vi "Entrenamiento Fuerza 5.vi"(8 "error in (no error)":errorcluster) -> (0 "error out":errorcluster)   [LabVIEW 2014]
panel:
  out "Label":string
  out "Master":bool
  out "element":T1
  in  "Master":bool
  out "OK":bool
  out "error out 2":errorcluster
  in  "Puerto Serial":refnum<visa-resource-name>="COM25"
  in  "index":i32
  out "size(s)":i32
  out "Decorations[]":refnum<vi>[](array[refnum])
  out "Boolean":bool
  out "Impulso":string
  out "Tiempo Restante":string
  out "Tiempo Transcurrido":string
  in  "Start":bool
  in  "Impulso":bool
  in  "Reset":bool
  in  "Back":bool
  in  "Help":bool
  in  "Slider":i32(slide) scale=0.0..100.0
  out "Horizontal Graduated Bar":i16(slide) scale=0.0..100.0
  in  "Remove Button":bool
  in  "Add Button":bool
  out "Opcional %":string="0%"
  in  "Opcional Bool":bool
  out "Biceps %":string="0%"
  in  "Biceps Bool":bool
  out "Pectorales %":string="0%"
  in  "Pectorales Bool":bool
  out "Trapecio %":string="0%"
  in  "Trapecio Bool":bool
  out "Dorsales %":string="0%"
  in  "Dorsales Bool":bool
  out "Lumbares %":string="0%"
  in  "Lumbares Bool":bool
  out "Abdomen %":string="0%"
  in  "Abdomen Bool":bool
  out "Gluteos %":string="0%"
  in  "Gluteos Bool":bool
  out "Isquiotibiales %":string="0%"
  in  "Isquiotibiales Bool":bool
  in  "Stop":bool
  out "Cuadríceps %":string="0%"
  in  "Cuadriceps Bool":bool
  out "date/time string":string="22/08/2015 01:25:29 a. m."
  # "Entrenamiento de Fuerza"
  # "Presentación"
  # "Seg"
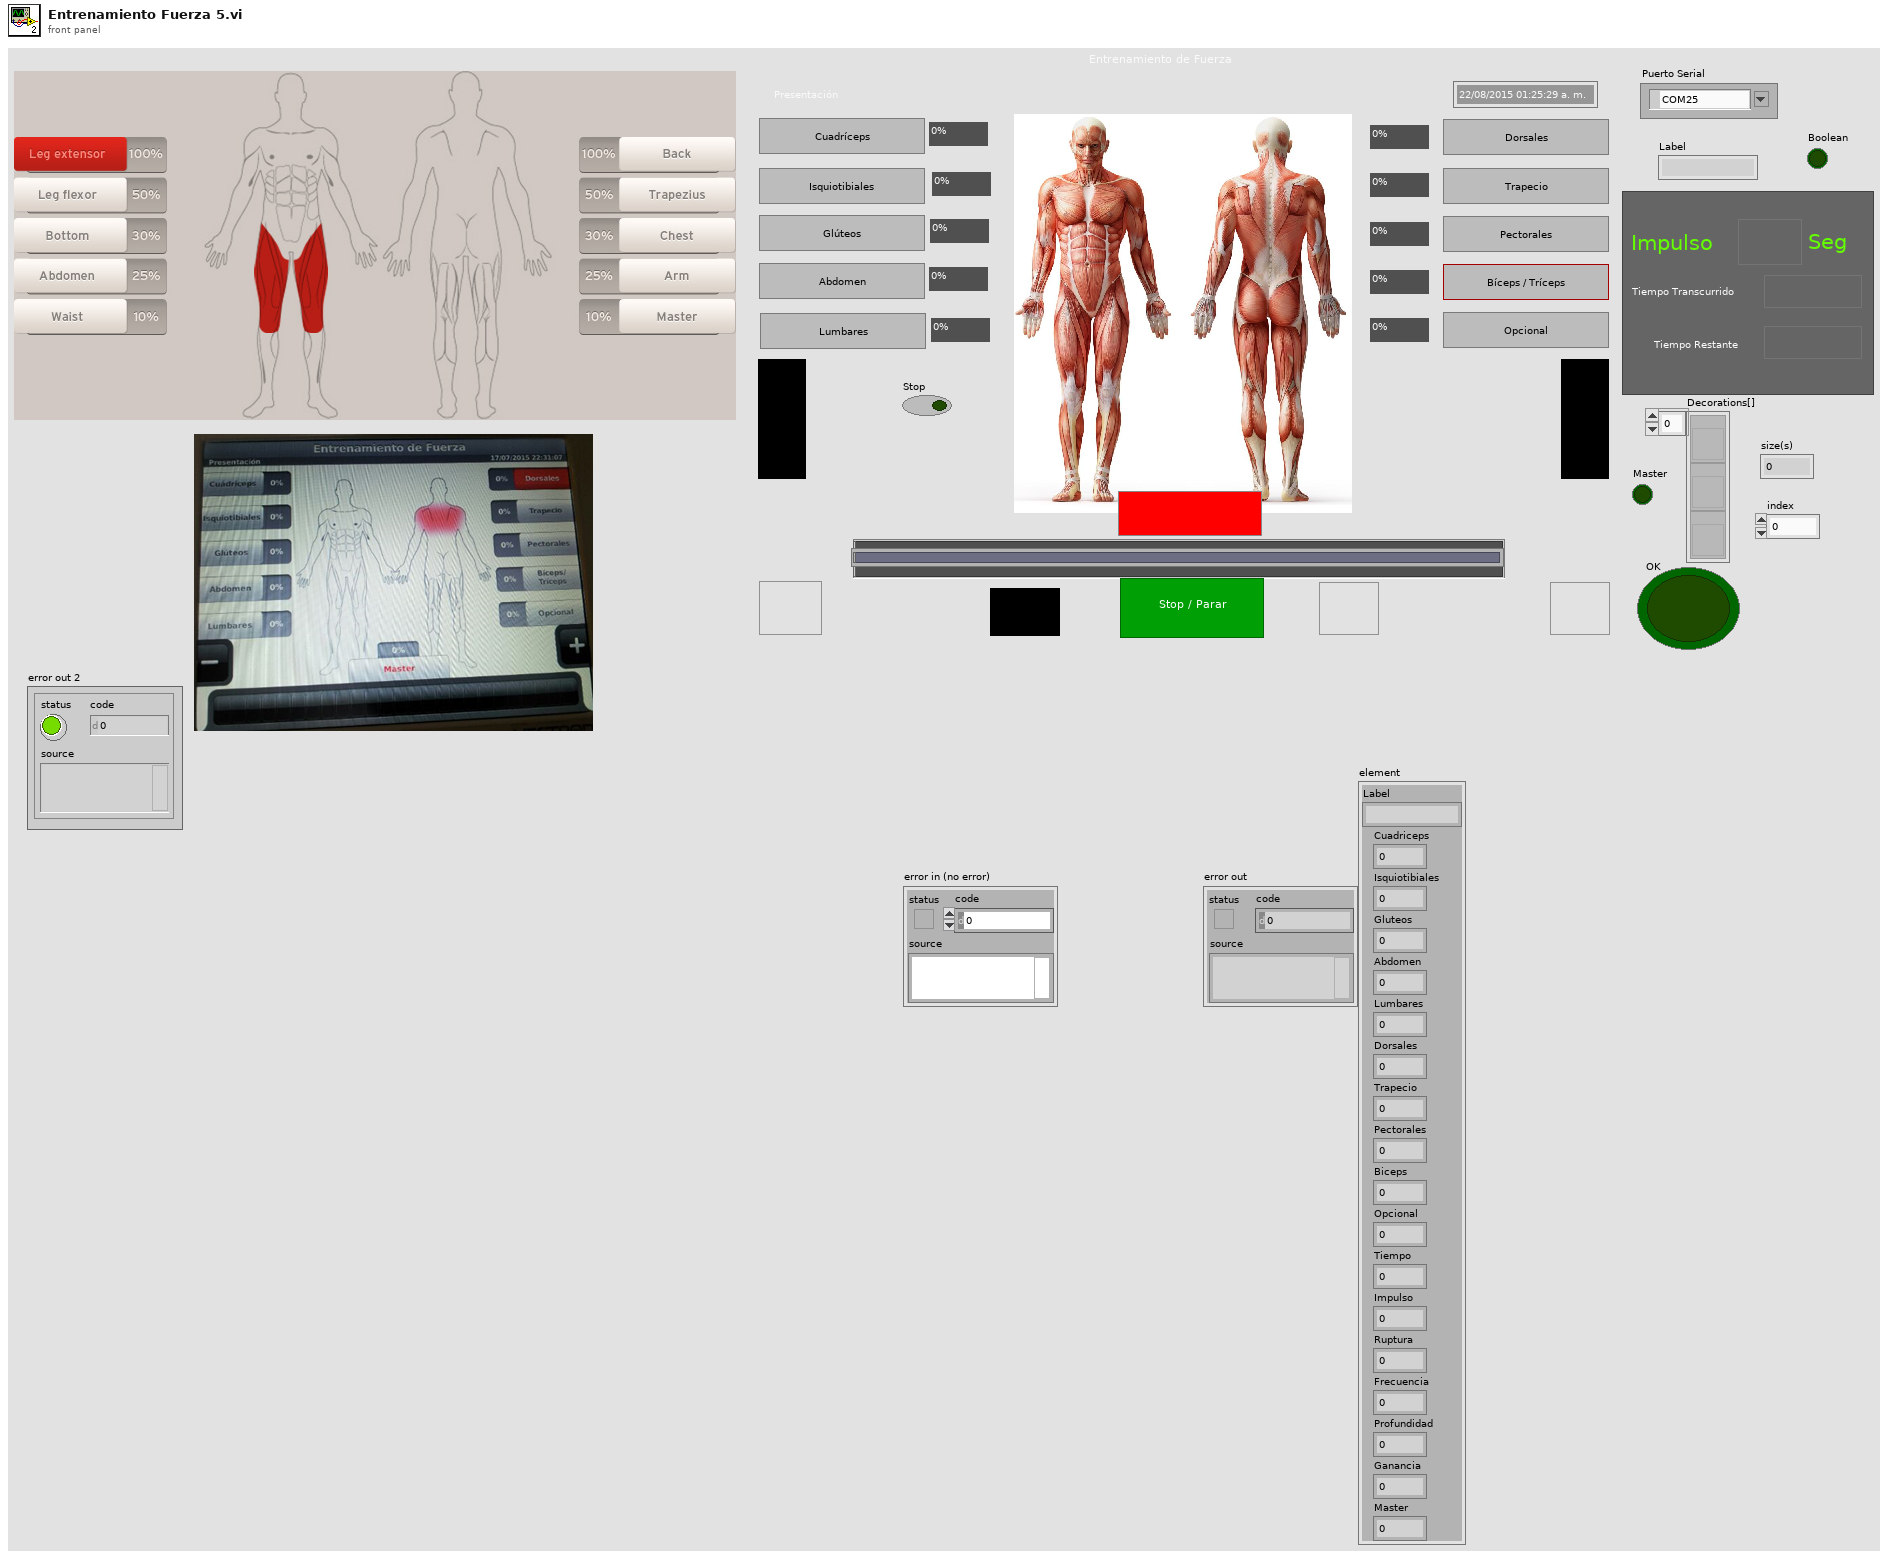
[diagram p1: front panel]
types:
  T1 = cluster{"Label":string, "Cuadriceps":i32, "Isquiotibiales":i32, "Gluteos":i32, "Abdomen":i32, "Lumbares":i32, "Dorsales":i32, "Trapecio":i32, "Pectorales":i32, "Biceps":i32, "Opcional":i32, "Tiempo":i32, "Impulso":i32, "Ruptura":i32, "Frecuencia":i32, "Profundidad":i32, "Ganancia":dbl, "Master":i32}
  T2 = cluster{"Boolean Text.Text Colors:Text Color":u32, u32}
  T3 = cluster{u32, "Boolean Text.Text Colors:Text Color":u32}
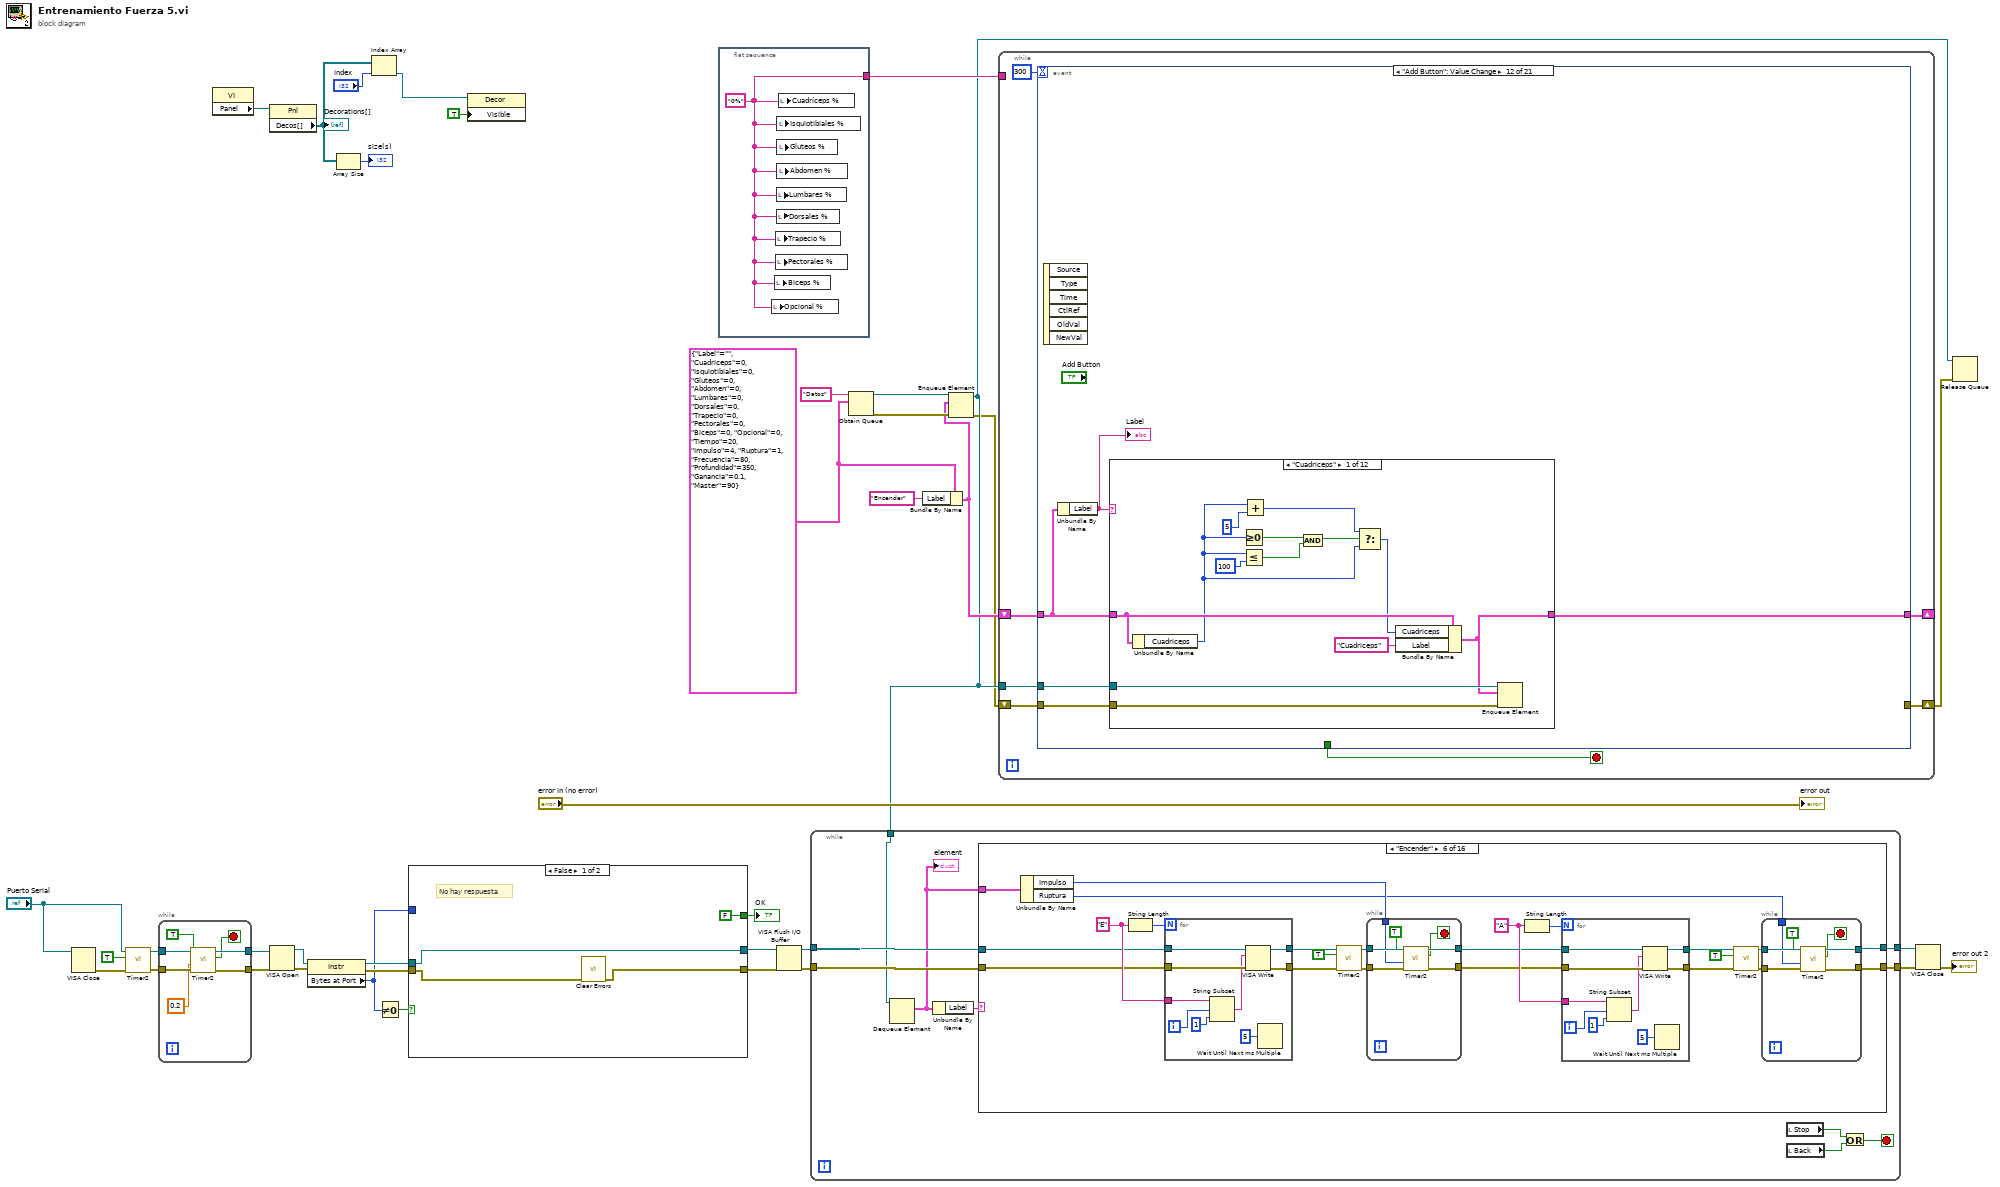
[diagram p0: block diagram]
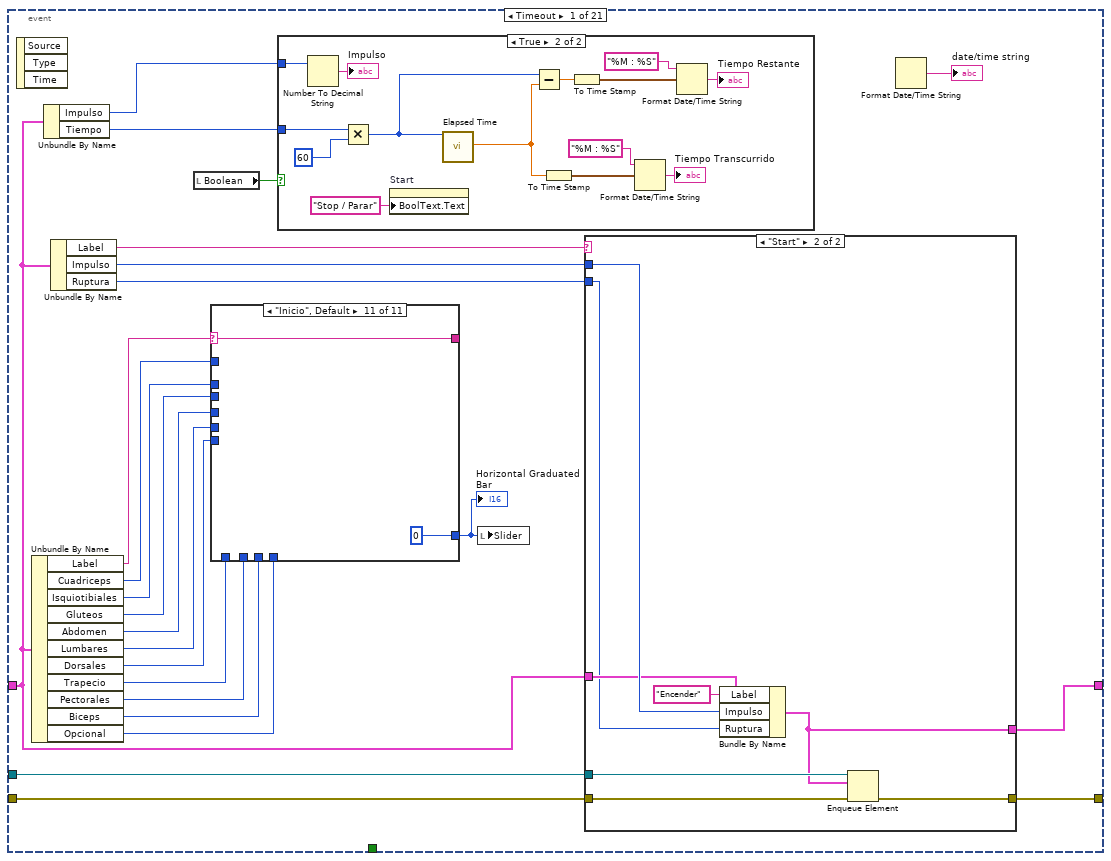
[diagram p2: hidden frame]
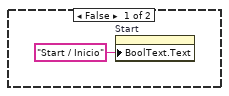
[diagram p4: hidden frame]
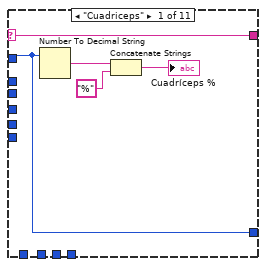
[diagram p5: hidden frame]
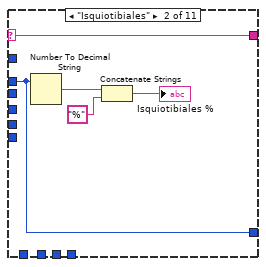
[diagram p6: hidden frame]
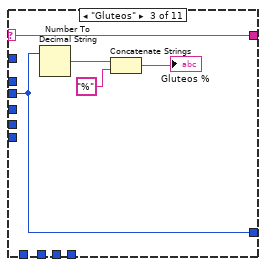
[diagram p7: hidden frame]
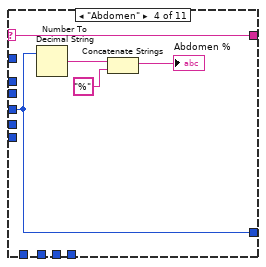
[diagram p8: hidden frame]
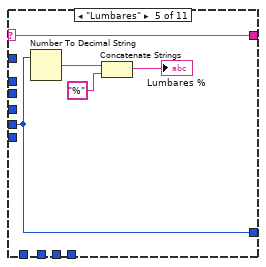
[diagram p9: hidden frame]
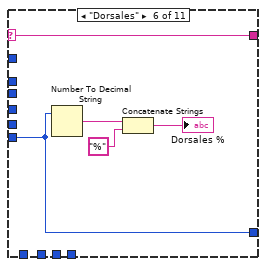
[diagram p10: hidden frame]
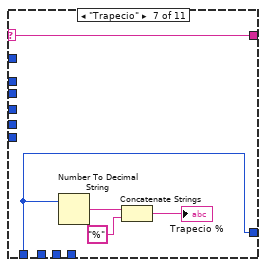
[diagram p11: hidden frame]
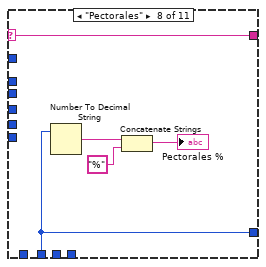
[diagram p12: hidden frame]
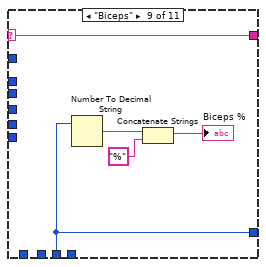
[diagram p13: hidden frame]
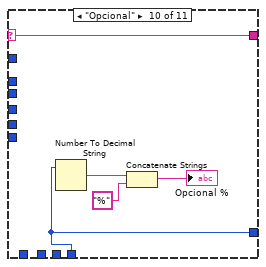
[diagram p14: hidden frame]
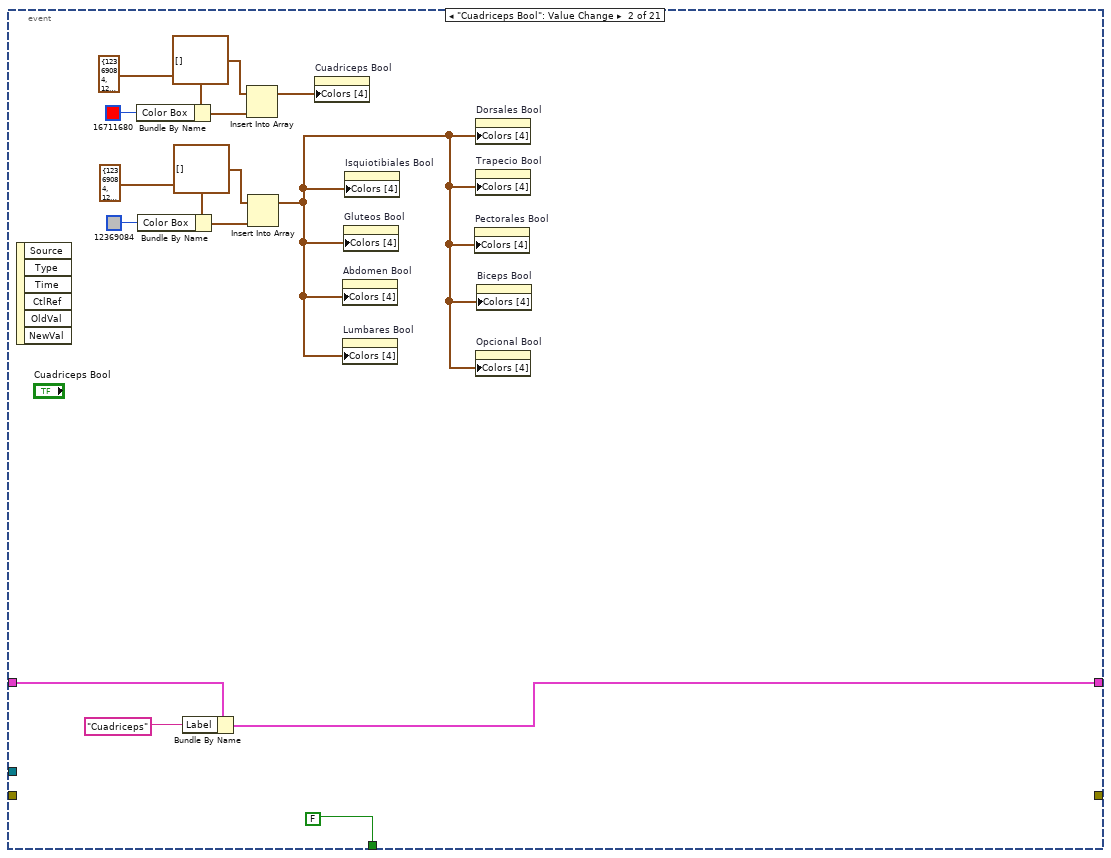
[diagram p15: hidden frame]
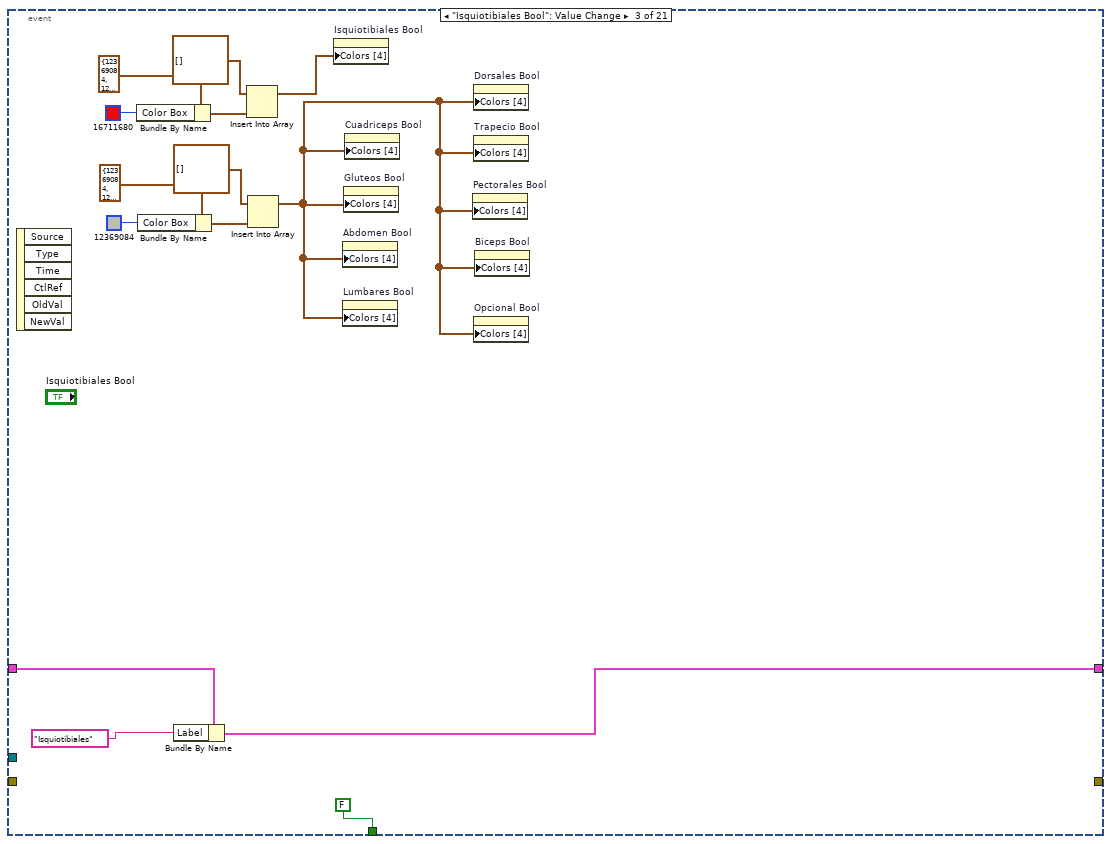
[diagram p16: hidden frame]
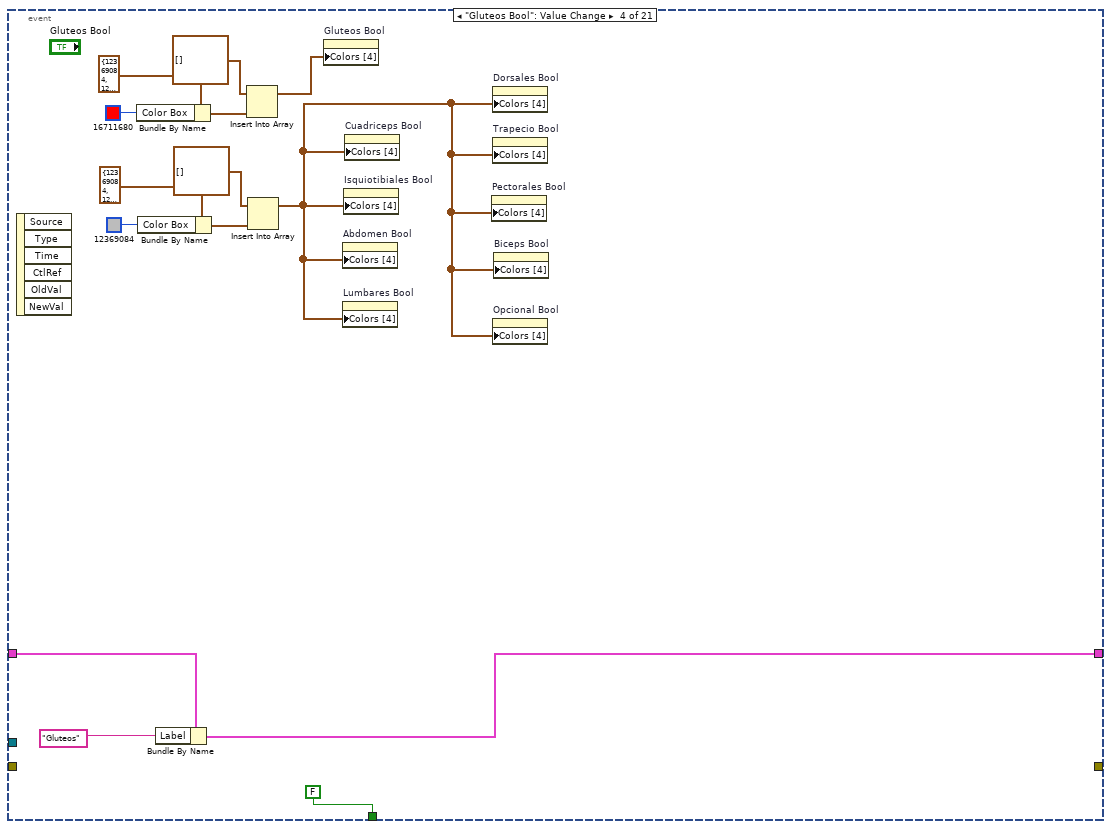
[diagram p17: hidden frame]
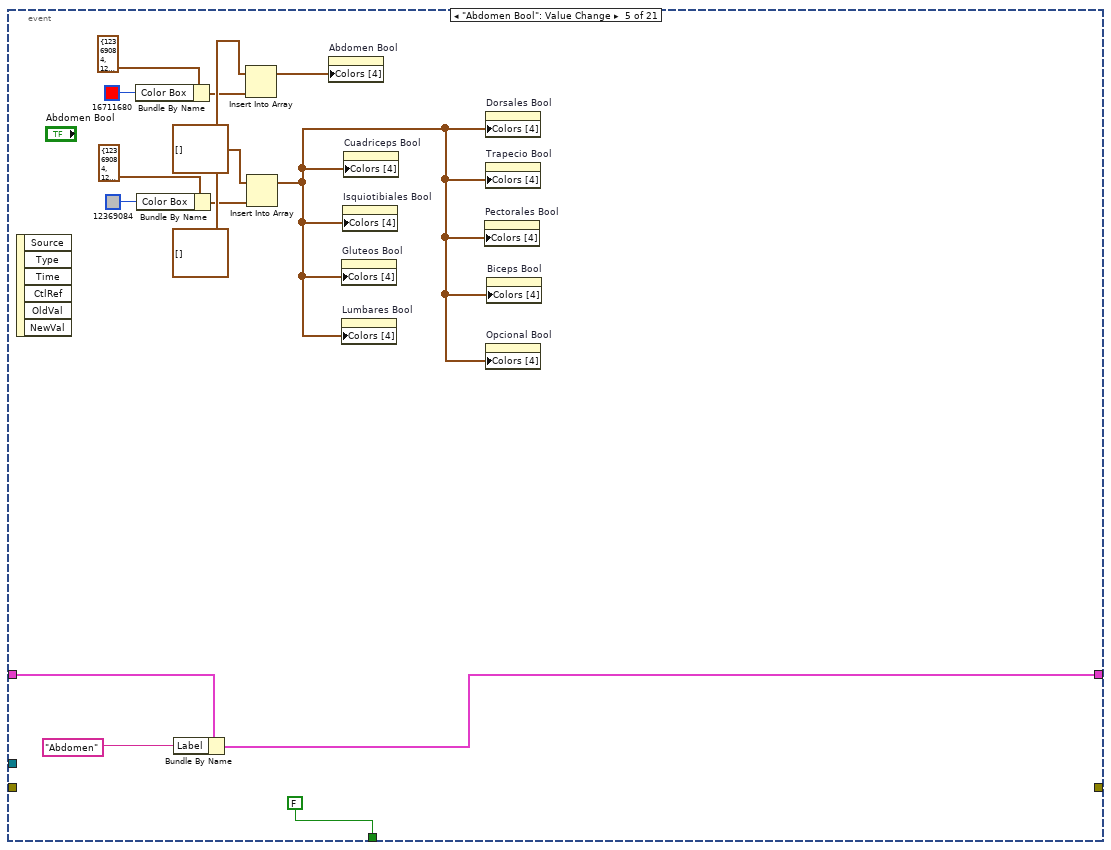
[diagram p18: hidden frame]
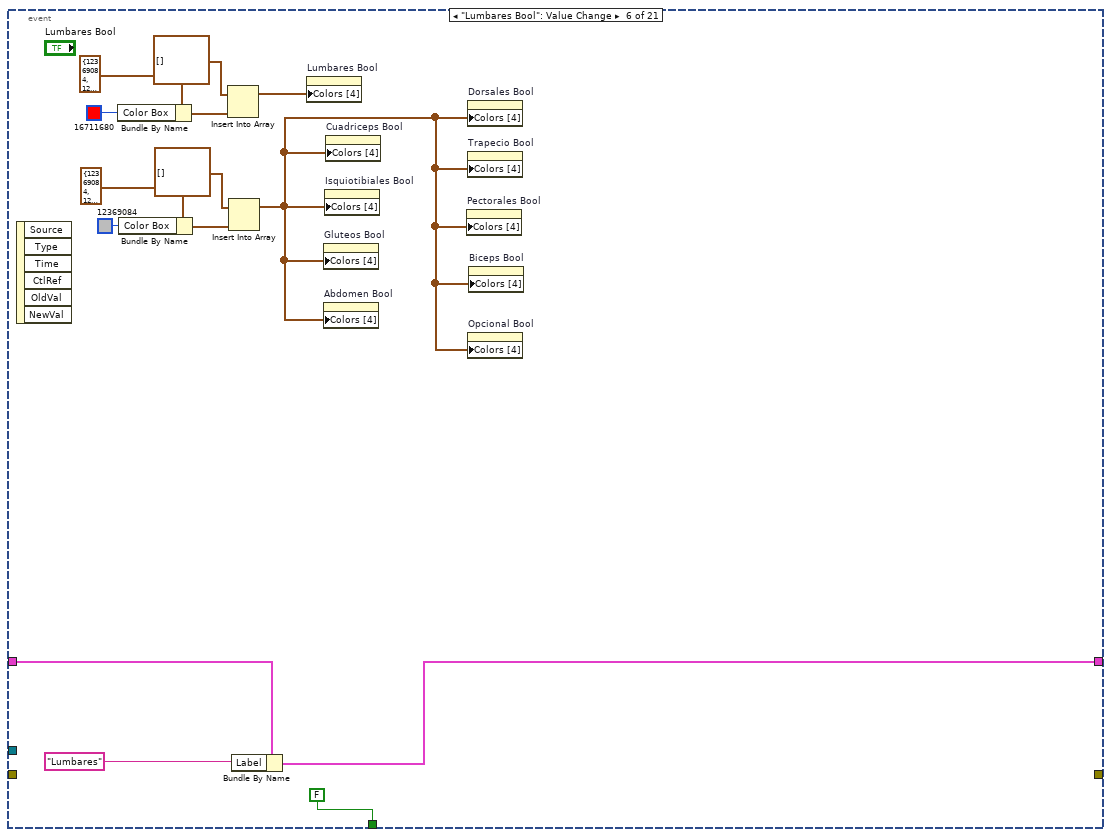
[diagram p19: hidden frame]
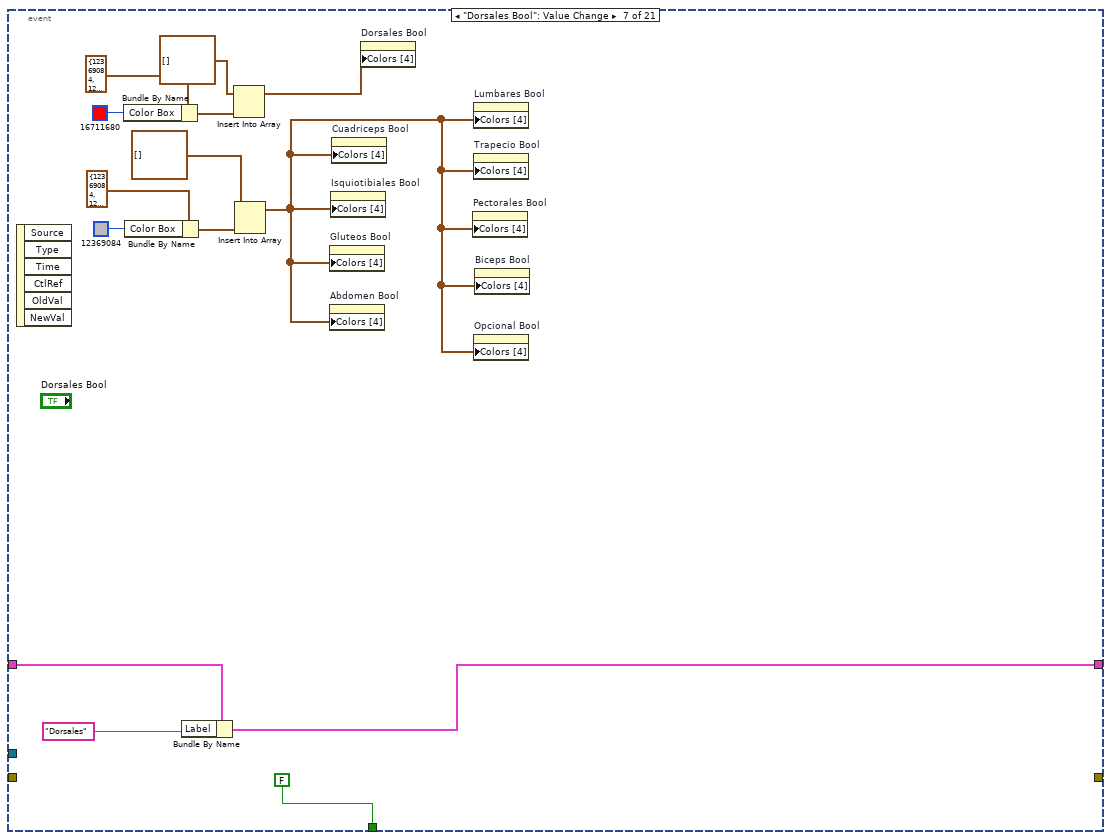
[diagram p20: hidden frame]
diagram:
  w7 = T1 {"Label"="", "Cuadriceps"=0, "Isquiotibiales"=0, "Gluteos"=0, "Abdomen"=0, "Lumbares"=0, "Dorsales"=0, "Trapecio"=0, "Pectorales"=0, "Biceps"=0, "Opcional"=0, "Tiempo"=20, "Impulso"=4, "Ruptura"=1, "Frecuencia"=80, "Profundidad"=350, "Ganancia"=0.1, "Master"=90}
  n1 = VISA Close(VISA resource name="Puerto Serial") -> (error out=w27:errorcluster)  [unwired: 1 in]
  n2 = call "Timer2.vi"("error in (no error)"=w27, "Reset"=TRUE) -> ("error out"=w26:errorcluster)  [unwired: 7 in, 2 out]
  n3 = while {
    tunnel: w26 -> [w42]
    tunnel: "Puerto Serial" -> [w43]
    tunnel: [w43] -> w28
    tunnel: [w41] -> w24
    stop <- w40 stop-if-true
    n4 = call "Timer2.vi"("error in (no error)"=w42, "Time Target (s)"=0.2, "Pause"=TRUE) -> ("error out"=w41:errorcluster, "Time has Elapsed"=w40:bool)  [unwired: 6 in, 1 out]
  }
  n5 = property class="VI"() -> ("Panel"=w36:refnum<vi>)  [unwired: 2 in, 2 out]
  n6 = property class="Pnl"(reference=w36) -> ("Decos[]"=w33:refnum<vi>[])  [unwired: 1 in, 2 out]
  "Decorations[]" <- w33
  n7 = VISA Open(error in (no error)=w24, VISA resource name=w28) -> (VISA resource name=w13:refnum<visa-resource-name>, error out=w17:errorcluster)  [unwired: 3 in]
  n8 = property class="Instr"(reference=w13, error in=w17) -> (reference out=w22:refnum<visa-resource-name>, error out=w23:errorcluster, "Bytes at Port"=w20:u32)
  n9 = Array Size(array=w33) -> (size(s)=→"size(s)":i32)
  n10 = Index Array(array=w33, index="index") -> (element=w32:refnum<vi>)
  n11 = Not Equal To 0?(x=w20) -> (x != 0?=w21:bool)
  n12 = case shown="False" w21 {
    tunnel: w23 -> [w45 w55]
    tunnel: w22 -> [w47 w54]
    tunnel: w20 -> [_ w53]
    tunnel: [w47 w51] -> w18
    tunnel: [w44 w50] -> w19
    tunnel: [FALSE w49] -> w14
    frame False {
      # "No hay respuesta"
      n13 = call <vilib>:"Clear Errors.vi"("error in (no error)"=w45) -> ("error out"=w44:errorcluster)  [unwired: 5 in, 1 out]
    }
    frame True {
      # "Recibe Datos de Respuesta"
      n14 = for {
        N: w53 -> [_]
        tunnel: w55 -> [w64]
        tunnel: w54 -> [w63]
        shift-right: [w58] -> w48
        shift-left: "" -> [w62]
        tunnel: [w61] -> w50
        tunnel: [w60] -> w51
        n15 = VISA Read(VISA resource name=w63, byte count=u32 1, error in (no error)=w64) -> (VISA resource name out=w60:refnum<visa-resource-name>, read buffer=w57:string, error out=w61:errorcluster)  [unwired: 1 out]
        n16 = Concatenate Strings(w62, w57) -> (w58:string)
        n17 = Wait Until Next ms Multiple(millisecond multiple=u32 1) -> ()  [unwired: 1 out]
      }
      n18 = Equal?(x=w48, y="OK") -> (x = y?=w49:bool)
    }
  }
  "OK" <- w14
  n19 = property class="Decor"(reference=w32, "Visible"=TRUE) -> ()  [unwired: 1 in, 2 out]
  n20 = flat-sequence {
    tunnel: [w66] -> w12
    frame #0 {
      w66 = "0%" ("Cuadríceps %")
      n21 = local write "Opcional %"(w66) -> ()
      n22 = local write "Biceps %"(w66) -> ()
      n23 = local write "Trapecio %"(w66) -> ()
      n24 = local write "Pectorales %"(w66) -> ()
      n25 = local write "Lumbares %"(w66) -> ()
      n26 = local write "Dorsales %"(w66) -> ()
      n27 = local write "Isquiotibiales %"(w66) -> ()
      n28 = local write "Gluteos %"(w66) -> ()
      n29 = local write "Abdomen %"(w66) -> ()
      n30 = local write "Cuadríceps %"(w66) -> ()
    }
  }
  n31 = VISA Flush I/O Buffer(VISA resource name=w18, error in (no error)=w19) -> (VISA resource name out=w15:refnum<visa-resource-name>, error out=w16:errorcluster)  [unwired: 1 in]
  n32 = Obtain Queue(name (unnamed)="Datos", element data type=w7) -> (queue out=w8:refnum<queue>, error out=w9:errorcluster)  [unwired: 3 in, 1 out]
  n33 = Bundle By Name(cluster=w7, "Label"="Encender") -> (w5:T1)
  n34 = Enqueue Element(queue=w8, element=w5, error in (no error)=w9) -> (queue out=w4:refnum<queue>, error out=w2:errorcluster)  [unwired: 1 in, 1 out]
  n35 = while {
    tunnel: w15 -> [w76]
    tunnel: [w73] -> w10
    tunnel: w16 -> [w75]
    tunnel: [w74] -> w11
    tunnel: w4 -> [w67]
    stop <- w69 stop-if-true
    n36 = Dequeue Element(queue=w67) -> (element=w68:T1)  [unwired: 2 in, 3 out]
    "element" <- w68
    n37 = Unbundle By Name(w68) -> ("Label"=w72:string)
    n38 = case shown="\"Encender\"" w72 {
      tunnel: w76 -> [w77 w92 w146 w200 w252 w294 w355 w407 w459 w511 w563 w615 w667 w719 w771 w823]
      tunnel: w75 -> [w78 w91 w145 w199 w251 w293 w354 w406 w458 w510 w562 w614 w666 w718 w770 w822]
      tunnel: [w78 w90 w144 w198 w250 w296 w353 w405 w457 w509 w561 w613 w665 w717 w769 w821] -> w74
      tunnel: [w77 w89 w143 w197 w249 w295 w352 w404 w456 w508 w560 w612 w664 w716 w768 w820] -> w73
      tunnel: w68 -> [_ w81 w136 w190 w239 w311 w344 w396 w448 w500 w552 w604 w656 w708 w760 w812]
      frame "Inicio", Default {
      }
      frame "Frecuencia" {
        n39 = Unbundle By Name(w81) -> ("Frecuencia"=w82:i32)
        n40 = To Unsigned Byte Integer(number=w82) -> (unsigned 8bit integer=w80:u8)
        n41 = Build Array(w80) -> (w79:u8[])
        n42 = Byte Array To String(unsigned byte array=w79) -> (string=w84:string)
        n43 = Concatenate Strings("F", w84) -> (w83:string)
        n44 = String Length(string=w83) -> (length=w88:i32)
        n45 = for {
          N: w88 -> [_]
          tunnel: w91 -> [w130]
          tunnel: w92 -> [w129]
          tunnel: w83 -> [w126]
          tunnel: [w123] -> w86
          tunnel: [w122] -> w87
          i -> [w124]
          n46 = String Subset(string=w126, offset (0)=w124, length (rest)=1 ("length (rest)")) -> (substring=w127:string)
          n47 = VISA Write(VISA resource name=w129, write buffer=w127, error in (no error)=w130) -> (VISA resource name out=w122:refnum<visa-resource-name>, error out=w123:errorcluster)  [unwired: 1 out]
          n48 = Wait Until Next ms Multiple(millisecond multiple=u32 5) -> ()  [unwired: 1 out]
        }
        n49 = disable-structure shown="Disabled" {
          disable-tunnel: [w104 w120] -> w90
          disable-tunnel: [w103 w121] -> w89
          disable-tunnel: w87 -> [w98 w121]
          disable-tunnel: w86 -> [w94 w120]
          frame Disabled {
            n50 = call "Timer2.vi"("error in (no error)"=w94, "Reset"=TRUE) -> ("error out"=w93:errorcluster)  [unwired: 7 in, 2 out]
            n51 = while {
              tunnel: w98 -> [w110]
              tunnel: [w110] -> w97
              tunnel: [w108] -> w96
              tunnel: w93 -> [w109]
              stop <- w107 stop-if-true
              n52 = call "Timer2.vi"("error in (no error)"=w109, "Time Target (s)"=0.25, "Pause"=TRUE) -> ("error out"=w108:errorcluster, "Time has Elapsed"=w107:bool)  [unwired: 6 in, 1 out]
            }
            n53 = property class="Instr"(reference=w97, error in=w96) -> (reference out=w101:refnum<visa-resource-name>, error out=w100:errorcluster, "Bytes at Port"=w99:u32)
            n54 = for {
              N: w99 -> [_]
              tunnel: w100 -> [w118]
              tunnel: w101 -> [w117]
              shift-right: [w112] -> _
              shift-left: "" -> [w116]
              tunnel: [w115] -> w104
              tunnel: [w114] -> w103
              n55 = VISA Read(VISA resource name=w117, byte count=u32 1, error in (no error)=w118) -> (VISA resource name out=w114:refnum<visa-resource-name>, read buffer=w111:string, error out=w115:errorcluster)  [unwired: 1 out]
              n56 = Concatenate Strings(w116, w111) -> (w112:string)
              n57 = Wait Until Next ms Multiple(millisecond multiple=u32 5) -> ()  [unwired: 1 out]
            }
          }
          frame Enabled {
          }
        }
      }
      frame "Ganancia" {
        n58 = Unbundle By Name(w136) -> ("Ganancia"=w132:dbl)
        n59 = Multiply(x=w132, y=10.0) -> (x*y=w133:dbl)
        n60 = To Unsigned Byte Integer(number=w133) -> (unsigned 8bit integer=w135:u8)
        n61 = Build Array(w135) -> (w134:u8[])
        n62 = Byte Array To String(unsigned byte array=w134) -> (string=w138:string)
        n63 = Concatenate Strings("G", w138) -> (w137:string)
        n64 = String Length(string=w137) -> (length=w142:i32)
        n65 = for {
          N: w142 -> [_]
          tunnel: w145 -> [w184]
          tunnel: w146 -> [w183]
          tunnel: w137 -> [w180]
          tunnel: [w177] -> w140
          tunnel: [w176] -> w141
          i -> [w178]
          n66 = String Subset(string=w180, offset (0)=w178, length (rest)=1 ("length (rest)")) -> (substring=w181:string)
          n67 = VISA Write(VISA resource name=w183, write buffer=w181, error in (no error)=w184) -> (VISA resource name out=w176:refnum<visa-resource-name>, error out=w177:errorcluster)  [unwired: 1 out]
          n68 = Wait Until Next ms Multiple(millisecond multiple=u32 5) -> ()  [unwired: 1 out]
        }
        n69 = disable-structure shown="Disabled" {
          disable-tunnel: [w158 w174] -> w144
          disable-tunnel: [w157 w175] -> w143
          disable-tunnel: w141 -> [w152 w175]
          disable-tunnel: w140 -> [w148 w174]
          frame Disabled {
            n70 = call "Timer2.vi"("error in (no error)"=w148, "Reset"=TRUE) -> ("error out"=w147:errorcluster)  [unwired: 7 in, 2 out]
            n71 = while {
              tunnel: w152 -> [w164]
              tunnel: [w164] -> w151
              tunnel: [w162] -> w150
              tunnel: w147 -> [w163]
              stop <- w161 stop-if-true
              n72 = call "Timer2.vi"("error in (no error)"=w163, "Time Target (s)"=0.25, "Pause"=TRUE) -> ("error out"=w162:errorcluster, "Time has Elapsed"=w161:bool)  [unwired: 6 in, 1 out]
            }
            n73 = property class="Instr"(reference=w151, error in=w150) -> (reference out=w155:refnum<visa-resource-name>, error out=w154:errorcluster, "Bytes at Port"=w153:u32)
            n74 = for {
              N: w153 -> [_]
              tunnel: w154 -> [w172]
              tunnel: w155 -> [w171]
              shift-right: [w166] -> _
              shift-left: "" -> [w170]
              tunnel: [w169] -> w158
              tunnel: [w168] -> w157
              n75 = VISA Read(VISA resource name=w171, byte count=u32 1, error in (no error)=w172) -> (VISA resource name out=w168:refnum<visa-resource-name>, read buffer=w165:string, error out=w169:errorcluster)  [unwired: 1 out]
              n76 = Concatenate Strings(w170, w165) -> (w166:string)
              n77 = Wait Until Next ms Multiple(millisecond multiple=u32 5) -> ()  [unwired: 1 out]
            }
          }
          frame Enabled {
          }
        }
      }
      frame "Impulso" {
        n78 = Unbundle By Name(w190) -> ("Profundidad"=w187:i32)
        n79 = To Unsigned Word Integer(number=w187) -> (unsigned 16bit integer=w186:u16)
        n80 = Split Number(x=w186) -> (hi(x)=w189:u8, lo(x)=w188:u8)
        n81 = Build Array(w189, w188) -> (w185:u8[])
        n82 = Byte Array To String(unsigned byte array=w185) -> (string=w192:string)
        n83 = Concatenate Strings("P", w192) -> (w191:string)
        n84 = String Length(string=w191) -> (length=w196:i32)
        n85 = for {
          N: w196 -> [_]
          tunnel: w199 -> [w238]
          tunnel: w200 -> [w237]
          tunnel: w191 -> [w234]
          tunnel: [w231] -> w194
          tunnel: [w230] -> w195
          i -> [w232]
          n86 = String Subset(string=w234, offset (0)=w232, length (rest)=1 ("length (rest)")) -> (substring=w235:string)
          n87 = VISA Write(VISA resource name=w237, write buffer=w235, error in (no error)=w238) -> (VISA resource name out=w230:refnum<visa-resource-name>, error out=w231:errorcluster)  [unwired: 1 out]
          n88 = Wait Until Next ms Multiple(millisecond multiple=u32 5) -> ()  [unwired: 1 out]
        }
        n89 = disable-structure shown="Disabled" {
          disable-tunnel: [w212 w228] -> w198
          disable-tunnel: [w211 w229] -> w197
          disable-tunnel: w195 -> [w206 w229]
          disable-tunnel: w194 -> [w202 w228]
          frame Disabled {
            n90 = call "Timer2.vi"("error in (no error)"=w202, "Reset"=TRUE) -> ("error out"=w201:errorcluster)  [unwired: 7 in, 2 out]
            n91 = while {
              tunnel: w206 -> [w218]
              tunnel: [w218] -> w205
              tunnel: [w216] -> w204
              tunnel: w201 -> [w217]
              stop <- w215 stop-if-true
              n92 = call "Timer2.vi"("error in (no error)"=w217, "Time Target (s)"=0.25, "Pause"=TRUE) -> ("error out"=w216:errorcluster, "Time has Elapsed"=w215:bool)  [unwired: 6 in, 1 out]
            }
            n93 = property class="Instr"(reference=w205, error in=w204) -> (reference out=w209:refnum<visa-resource-name>, error out=w208:errorcluster, "Bytes at Port"=w207:u32)
            n94 = for {
              N: w207 -> [_]
              tunnel: w208 -> [w226]
              tunnel: w209 -> [w225]
              shift-right: [w220] -> _
              shift-left: "" -> [w224]
              tunnel: [w223] -> w212
              tunnel: [w222] -> w211
              n95 = VISA Read(VISA resource name=w225, byte count=u32 1, error in (no error)=w226) -> (VISA resource name out=w222:refnum<visa-resource-name>, read buffer=w219:string, error out=w223:errorcluster)  [unwired: 1 out]
              n96 = Concatenate Strings(w224, w219) -> (w220:string)
              n97 = Wait Until Next ms Multiple(millisecond multiple=u32 5) -> ()  [unwired: 1 out]
            }
          }
          frame Enabled {
          }
        }
      }
      frame "Master" {
        n98 = Unbundle By Name(w239) -> ("Master"=w242:i32)
        n99 = To Unsigned Byte Integer(number=w242) -> (unsigned 8bit integer=w241:u8)
        n100 = Build Array(w241) -> (w240:u8[])
        n101 = Byte Array To String(unsigned byte array=w240) -> (string=w244:string)
        n102 = Concatenate Strings("M", w244) -> (w243:string)
        n103 = String Length(string=w243) -> (length=w248:i32)
        n104 = for {
          N: w248 -> [_]
          tunnel: w251 -> [w290]
          tunnel: w252 -> [w289]
          tunnel: w243 -> [w286]
          tunnel: [w283] -> w246
          tunnel: [w282] -> w247
          i -> [w284]
          n105 = String Subset(string=w286, offset (0)=w284, length (rest)=1 ("length (rest)")) -> (substring=w287:string)
          n106 = VISA Write(VISA resource name=w289, write buffer=w287, error in (no error)=w290) -> (VISA resource name out=w282:refnum<visa-resource-name>, error out=w283:errorcluster)  [unwired: 1 out]
          n107 = Wait Until Next ms Multiple(millisecond multiple=u32 5) -> ()  [unwired: 1 out]
        }
        n108 = disable-structure shown="Disabled" {
          disable-tunnel: [w264 w280] -> w250
          disable-tunnel: [w263 w281] -> w249
          disable-tunnel: w247 -> [w258 w281]
          disable-tunnel: w246 -> [w254 w280]
          frame Disabled {
            n109 = call "Timer2.vi"("error in (no error)"=w254, "Reset"=TRUE) -> ("error out"=w253:errorcluster)  [unwired: 7 in, 2 out]
            n110 = while {
              tunnel: w258 -> [w270]
              tunnel: [w270] -> w257
              tunnel: [w268] -> w256
              tunnel: w253 -> [w269]
              stop <- w267 stop-if-true
              n111 = call "Timer2.vi"("error in (no error)"=w269, "Time Target (s)"=0.25, "Pause"=TRUE) -> ("error out"=w268:errorcluster, "Time has Elapsed"=w267:bool)  [unwired: 6 in, 1 out]
            }
            n112 = property class="Instr"(reference=w257, error in=w256) -> (reference out=w261:refnum<visa-resource-name>, error out=w260:errorcluster, "Bytes at Port"=w259:u32)
            n113 = for {
              N: w259 -> [_]
              tunnel: w260 -> [w278]
              tunnel: w261 -> [w277]
              shift-right: [w272] -> _
              shift-left: "" -> [w276]
              tunnel: [w275] -> w264
              tunnel: [w274] -> w263
              n114 = VISA Read(VISA resource name=w277, byte count=u32 1, error in (no error)=w278) -> (VISA resource name out=w274:refnum<visa-resource-name>, read buffer=w271:string, error out=w275:errorcluster)  [unwired: 1 out]
              n115 = Concatenate Strings(w276, w271) -> (w272:string)
              n116 = Wait Until Next ms Multiple(millisecond multiple=u32 5) -> ()  [unwired: 1 out]
            }
          }
          frame Enabled {
          }
        }
      }
      frame "Encender" {
        w301 = "A"
        w307 = "E"
        n117 = Unbundle By Name(w311) -> ("Impulso"=w292:i32, "Ruptura"=w291:i32)
        n118 = String Length(string=w307) -> (length=w310:i32)
        n119 = for {
          N: w310 -> [_]
          tunnel: w293 -> [w341]
          tunnel: w294 -> [w340]
          tunnel: w307 -> [w337]
          tunnel: [w334] -> w308
          tunnel: [w333] -> w309
          i -> [w335]
          n120 = String Subset(string=w337, offset (0)=w335, length (rest)=1 ("length (rest)")) -> (substring=w338:string)
          n121 = VISA Write(VISA resource name=w340, write buffer=w338, error in (no error)=w341) -> (VISA resource name out=w333:refnum<visa-resource-name>, error out=w334:errorcluster)  [unwired: 1 out]
          n122 = Wait Until Next ms Multiple(millisecond multiple=u32 5) -> ()  [unwired: 1 out]
        }
        n123 = call "Timer2.vi"("error in (no error)"=w308, "Reset"=TRUE) -> ("error out"=w305:errorcluster)  [unwired: 7 in, 2 out]
        n124 = while {
          tunnel: w309 -> [w332]
          tunnel: [w332] -> w298
          tunnel: [w330] -> w297
          tunnel: w305 -> [w331]
          tunnel: w292 -> [w327]
          stop <- w329 stop-if-true
          n125 = call "Timer2.vi"("error in (no error)"=w331, "Time Target (s)"=w327, "Pause"=TRUE) -> ("error out"=w330:errorcluster, "Time has Elapsed"=w329:bool)  [unwired: 6 in, 1 out]
        }
        n126 = String Length(string=w301) -> (length=w304:i32)
        n127 = for {
          N: w304 -> [_]
          tunnel: w297 -> [w326]
          tunnel: w298 -> [w325]
          tunnel: w301 -> [w322]
          tunnel: [w319] -> w302
          tunnel: [w318] -> w303
          i -> [w320]
          n128 = String Subset(string=w322, offset (0)=w320, length (rest)=1 ("length (rest)")) -> (substring=w323:string)
          n129 = VISA Write(VISA resource name=w325, write buffer=w323, error in (no error)=w326) -> (VISA resource name out=w318:refnum<visa-resource-name>, error out=w319:errorcluster)  [unwired: 1 out]
          n130 = Wait Until Next ms Multiple(millisecond multiple=u32 5) -> ()  [unwired: 1 out]
        }
        n131 = call "Timer2.vi"("error in (no error)"=w302, "Reset"=TRUE) -> ("error out"=w299:errorcluster)  [unwired: 7 in, 2 out]
        n132 = while {
          tunnel: w303 -> [w317]
          tunnel: [w317] -> w295
          tunnel: [w315] -> w296
          tunnel: w299 -> [w316]
          tunnel: w291 -> [w312]
          stop <- w314 stop-if-true
          n133 = call "Timer2.vi"("error in (no error)"=w316, "Time Target (s)"=w312, "Pause"=TRUE) -> ("error out"=w315:errorcluster, "Time has Elapsed"=w314:bool)  [unwired: 6 in, 1 out]
        }
      }
      frame "Cuadriceps" {
        n134 = Unbundle By Name(w344) -> ("Cuadriceps"=w342:i32)
        n135 = To Unsigned Byte Integer(number=w342) -> (unsigned 8bit integer=w343:u8)
        n136 = Build Array(w343) -> (w348:u8[])
        n137 = Byte Array To String(unsigned byte array=w348) -> (string=w346:string)
        n138 = Concatenate Strings("1", w346) -> (w345:string)
        n139 = String Length(string=w345) -> (length=w351:i32)
        n140 = for {
          N: w351 -> [_]
          tunnel: w354 -> [w393]
          tunnel: w355 -> [w392]
          tunnel: w345 -> [w389]
          tunnel: [w386] -> w349
          tunnel: [w385] -> w350
          i -> [w387]
          n141 = String Subset(string=w389, offset (0)=w387, length (rest)=1 ("length (rest)")) -> (substring=w390:string)
          n142 = VISA Write(VISA resource name=w392, write buffer=w390, error in (no error)=w393) -> (VISA resource name out=w385:refnum<visa-resource-name>, error out=w386:errorcluster)  [unwired: 1 out]
          n143 = Wait Until Next ms Multiple(millisecond multiple=u32 5) -> ()  [unwired: 1 out]
        }
        n144 = disable-structure shown="Disabled" {
          disable-tunnel: [w367 w383] -> w353
          disable-tunnel: [w366 w384] -> w352
          disable-tunnel: w350 -> [w361 w384]
          disable-tunnel: w349 -> [w357 w383]
          frame Disabled {
            n145 = call "Timer2.vi"("error in (no error)"=w357, "Reset"=TRUE) -> ("error out"=w356:errorcluster)  [unwired: 7 in, 2 out]
            n146 = while {
              tunnel: w361 -> [w373]
              tunnel: [w373] -> w360
              tunnel: [w371] -> w359
              tunnel: w356 -> [w372]
              stop <- w370 stop-if-true
              n147 = call "Timer2.vi"("error in (no error)"=w372, "Time Target (s)"=0.25, "Pause"=TRUE) -> ("error out"=w371:errorcluster, "Time has Elapsed"=w370:bool)  [unwired: 6 in, 1 out]
            }
            n148 = property class="Instr"(reference=w360, error in=w359) -> (reference out=w364:refnum<visa-resource-name>, error out=w363:errorcluster, "Bytes at Port"=w362:u32)
            n149 = for {
              N: w362 -> [_]
              tunnel: w363 -> [w381]
              tunnel: w364 -> [w380]
              shift-right: [w375] -> _
              shift-left: "" -> [w379]
              tunnel: [w378] -> w367
              tunnel: [w377] -> w366
              n150 = VISA Read(VISA resource name=w380, byte count=u32 1, error in (no error)=w381) -> (VISA resource name out=w377:refnum<visa-resource-name>, read buffer=w374:string, error out=w378:errorcluster)  [unwired: 1 out]
              n151 = Concatenate Strings(w379, w374) -> (w375:string)
              n152 = Wait Until Next ms Multiple(millisecond multiple=u32 5) -> ()  [unwired: 1 out]
            }
          }
          frame Enabled {
          }
        }
      }
      frame "Isquiotibiales" {
        n153 = Unbundle By Name(w396) -> ("Isquiotibiales"=w394:i32)
        n154 = To Unsigned Byte Integer(number=w394) -> (unsigned 8bit integer=w395:u8)
        n155 = Build Array(w395) -> (w400:u8[])
        n156 = Byte Array To String(unsigned byte array=w400) -> (string=w398:string)
        n157 = Concatenate Strings("2", w398) -> (w397:string)
        n158 = String Length(string=w397) -> (length=w403:i32)
        n159 = for {
          N: w403 -> [_]
          tunnel: w406 -> [w445]
          tunnel: w407 -> [w444]
          tunnel: w397 -> [w441]
          tunnel: [w438] -> w401
          tunnel: [w437] -> w402
          i -> [w439]
          n160 = String Subset(string=w441, offset (0)=w439, length (rest)=1 ("length (rest)")) -> (substring=w442:string)
          n161 = VISA Write(VISA resource name=w444, write buffer=w442, error in (no error)=w445) -> (VISA resource name out=w437:refnum<visa-resource-name>, error out=w438:errorcluster)  [unwired: 1 out]
          n162 = Wait Until Next ms Multiple(millisecond multiple=u32 5) -> ()  [unwired: 1 out]
        }
        n163 = disable-structure shown="Disabled" {
          disable-tunnel: [w419 w435] -> w405
          disable-tunnel: [w418 w436] -> w404
          disable-tunnel: w402 -> [w413 w436]
          disable-tunnel: w401 -> [w409 w435]
          frame Disabled {
            n164 = call "Timer2.vi"("error in (no error)"=w409, "Reset"=TRUE) -> ("error out"=w408:errorcluster)  [unwired: 7 in, 2 out]
            n165 = while {
              tunnel: w413 -> [w425]
              tunnel: [w425] -> w412
              tunnel: [w423] -> w411
              tunnel: w408 -> [w424]
              stop <- w422 stop-if-true
              n166 = call "Timer2.vi"("error in (no error)"=w424, "Time Target (s)"=0.25, "Pause"=TRUE) -> ("error out"=w423:errorcluster, "Time has Elapsed"=w422:bool)  [unwired: 6 in, 1 out]
            }
            n167 = property class="Instr"(reference=w412, error in=w411) -> (reference out=w416:refnum<visa-resource-name>, error out=w415:errorcluster, "Bytes at Port"=w414:u32)
            n168 = for {
              N: w414 -> [_]
              tunnel: w415 -> [w433]
              tunnel: w416 -> [w432]
              shift-right: [w427] -> _
              shift-left: "" -> [w431]
              tunnel: [w430] -> w419
              tunnel: [w429] -> w418
              n169 = VISA Read(VISA resource name=w432, byte count=u32 1, error in (no error)=w433) -> (VISA resource name out=w429:refnum<visa-resource-name>, read buffer=w426:string, error out=w430:errorcluster)  [unwired: 1 out]
              n170 = Concatenate Strings(w431, w426) -> (w427:string)
              n171 = Wait Until Next ms Multiple(millisecond multiple=u32 5) -> ()  [unwired: 1 out]
            }
          }
          frame Enabled {
          }
        }
      }
      frame "Gluteos" {
        n172 = Unbundle By Name(w448) -> ("Gluteos"=w446:i32)
        n173 = To Unsigned Byte Integer(number=w446) -> (unsigned 8bit integer=w447:u8)
        n174 = Build Array(w447) -> (w452:u8[])
        n175 = Byte Array To String(unsigned byte array=w452) -> (string=w450:string)
        n176 = Concatenate Strings("3", w450) -> (w449:string)
        n177 = String Length(string=w449) -> (length=w455:i32)
        n178 = for {
          N: w455 -> [_]
          tunnel: w458 -> [w497]
          tunnel: w459 -> [w496]
          tunnel: w449 -> [w493]
          tunnel: [w490] -> w453
          tunnel: [w489] -> w454
          i -> [w491]
          n179 = String Subset(string=w493, offset (0)=w491, length (rest)=1 ("length (rest)")) -> (substring=w494:string)
          n180 = VISA Write(VISA resource name=w496, write buffer=w494, error in (no error)=w497) -> (VISA resource name out=w489:refnum<visa-resource-name>, error out=w490:errorcluster)  [unwired: 1 out]
          n181 = Wait Until Next ms Multiple(millisecond multiple=u32 5) -> ()  [unwired: 1 out]
        }
        n182 = disable-structure shown="Disabled" {
          disable-tunnel: [w471 w487] -> w457
          disable-tunnel: [w470 w488] -> w456
          disable-tunnel: w454 -> [w465 w488]
          disable-tunnel: w453 -> [w461 w487]
          frame Disabled {
            n183 = call "Timer2.vi"("error in (no error)"=w461, "Reset"=TRUE) -> ("error out"=w460:errorcluster)  [unwired: 7 in, 2 out]
            n184 = while {
              tunnel: w465 -> [w477]
              tunnel: [w477] -> w464
              tunnel: [w475] -> w463
              tunnel: w460 -> [w476]
              stop <- w474 stop-if-true
              n185 = call "Timer2.vi"("error in (no error)"=w476, "Time Target (s)"=0.25, "Pause"=TRUE) -> ("error out"=w475:errorcluster, "Time has Elapsed"=w474:bool)  [unwired: 6 in, 1 out]
            }
            n186 = property class="Instr"(reference=w464, error in=w463) -> (reference out=w468:refnum<visa-resource-name>, error out=w467:errorcluster, "Bytes at Port"=w466:u32)
            n187 = for {
              N: w466 -> [_]
              tunnel: w467 -> [w485]
              tunnel: w468 -> [w484]
              shift-right: [w479] -> _
              shift-left: "" -> [w483]
              tunnel: [w482] -> w471
              tunnel: [w481] -> w470
              n188 = VISA Read(VISA resource name=w484, byte count=u32 1, error in (no error)=w485) -> (VISA resource name out=w481:refnum<visa-resource-name>, read buffer=w478:string, error out=w482:errorcluster)  [unwired: 1 out]
              n189 = Concatenate Strings(w483, w478) -> (w479:string)
              n190 = Wait Until Next ms Multiple(millisecond multiple=u32 5) -> ()  [unwired: 1 out]
            }
          }
          frame Enabled {
          }
        }
      }
      frame "Abdomen" {
        n191 = Unbundle By Name(w500) -> ("Abdomen"=w498:i32)
        n192 = To Unsigned Byte Integer(number=w498) -> (unsigned 8bit integer=w499:u8)
        n193 = Build Array(w499) -> (w504:u8[])
        n194 = Byte Array To String(unsigned byte array=w504) -> (string=w502:string)
        n195 = Concatenate Strings("4", w502) -> (w501:string)
        n196 = String Length(string=w501) -> (length=w507:i32)
        n197 = for {
          N: w507 -> [_]
          tunnel: w510 -> [w549]
          tunnel: w511 -> [w548]
          tunnel: w501 -> [w545]
          tunnel: [w542] -> w505
          tunnel: [w541] -> w506
          i -> [w543]
          n198 = String Subset(string=w545, offset (0)=w543, length (rest)=1 ("length (rest)")) -> (substring=w546:string)
          n199 = VISA Write(VISA resource name=w548, write buffer=w546, error in (no error)=w549) -> (VISA resource name out=w541:refnum<visa-resource-name>, error out=w542:errorcluster)  [unwired: 1 out]
          n200 = Wait Until Next ms Multiple(millisecond multiple=u32 5) -> ()  [unwired: 1 out]
        }
        n201 = disable-structure shown="Disabled" {
          disable-tunnel: [w523 w539] -> w509
          disable-tunnel: [w522 w540] -> w508
          disable-tunnel: w506 -> [w517 w540]
          disable-tunnel: w505 -> [w513 w539]
          frame Disabled {
            n202 = call "Timer2.vi"("error in (no error)"=w513, "Reset"=TRUE) -> ("error out"=w512:errorcluster)  [unwired: 7 in, 2 out]
            n203 = while {
              tunnel: w517 -> [w529]
              tunnel: [w529] -> w516
              tunnel: [w527] -> w515
              tunnel: w512 -> [w528]
              stop <- w526 stop-if-true
              n204 = call "Timer2.vi"("error in (no error)"=w528, "Time Target (s)"=0.25, "Pause"=TRUE) -> ("error out"=w527:errorcluster, "Time has Elapsed"=w526:bool)  [unwired: 6 in, 1 out]
            }
            n205 = property class="Instr"(reference=w516, error in=w515) -> (reference out=w520:refnum<visa-resource-name>, error out=w519:errorcluster, "Bytes at Port"=w518:u32)
            n206 = for {
              N: w518 -> [_]
              tunnel: w519 -> [w537]
              tunnel: w520 -> [w536]
              shift-right: [w531] -> _
              shift-left: "" -> [w535]
              tunnel: [w534] -> w523
              tunnel: [w533] -> w522
              n207 = VISA Read(VISA resource name=w536, byte count=u32 1, error in (no error)=w537) -> (VISA resource name out=w533:refnum<visa-resource-name>, read buffer=w530:string, error out=w534:errorcluster)  [unwired: 1 out]
              n208 = Concatenate Strings(w535, w530) -> (w531:string)
              n209 = Wait Until Next ms Multiple(millisecond multiple=u32 5) -> ()  [unwired: 1 out]
            }
          }
          frame Enabled {
          }
        }
      }
      frame "Lumbares" {
        n210 = Unbundle By Name(w552) -> ("Lumbares"=w550:i32)
        n211 = To Unsigned Byte Integer(number=w550) -> (unsigned 8bit integer=w551:u8)
        n212 = Build Array(w551) -> (w556:u8[])
        n213 = Byte Array To String(unsigned byte array=w556) -> (string=w554:string)
        n214 = Concatenate Strings("5", w554) -> (w553:string)
        n215 = String Length(string=w553) -> (length=w559:i32)
        n216 = for {
          N: w559 -> [_]
          tunnel: w562 -> [w601]
          tunnel: w563 -> [w600]
          tunnel: w553 -> [w597]
          tunnel: [w594] -> w557
          tunnel: [w593] -> w558
          i -> [w595]
          n217 = String Subset(string=w597, offset (0)=w595, length (rest)=1 ("length (rest)")) -> (substring=w598:string)
          n218 = VISA Write(VISA resource name=w600, write buffer=w598, error in (no error)=w601) -> (VISA resource name out=w593:refnum<visa-resource-name>, error out=w594:errorcluster)  [unwired: 1 out]
          n219 = Wait Until Next ms Multiple(millisecond multiple=u32 5) -> ()  [unwired: 1 out]
        }
        n220 = disable-structure shown="Disabled" {
          disable-tunnel: [w575 w591] -> w561
          disable-tunnel: [w574 w592] -> w560
          disable-tunnel: w558 -> [w569 w592]
          disable-tunnel: w557 -> [w565 w591]
          frame Disabled {
            n221 = call "Timer2.vi"("error in (no error)"=w565, "Reset"=TRUE) -> ("error out"=w564:errorcluster)  [unwired: 7 in, 2 out]
            n222 = while {
              tunnel: w569 -> [w581]
              tunnel: [w581] -> w568
              tunnel: [w579] -> w567
              tunnel: w564 -> [w580]
              stop <- w578 stop-if-true
              n223 = call "Timer2.vi"("error in (no error)"=w580, "Time Target (s)"=0.25, "Pause"=TRUE) -> ("error out"=w579:errorcluster, "Time has Elapsed"=w578:bool)  [unwired: 6 in, 1 out]
            }
            n224 = property class="Instr"(reference=w568, error in=w567) -> (reference out=w572:refnum<visa-resource-name>, error out=w571:errorcluster, "Bytes at Port"=w570:u32)
            n225 = for {
              N: w570 -> [_]
              tunnel: w571 -> [w589]
              tunnel: w572 -> [w588]
              shift-right: [w583] -> _
              shift-left: "" -> [w587]
              tunnel: [w586] -> w575
              tunnel: [w585] -> w574
              n226 = VISA Read(VISA resource name=w588, byte count=u32 1, error in (no error)=w589) -> (VISA resource name out=w585:refnum<visa-resource-name>, read buffer=w582:string, error out=w586:errorcluster)  [unwired: 1 out]
              n227 = Concatenate Strings(w587, w582) -> (w583:string)
              n228 = Wait Until Next ms Multiple(millisecond multiple=u32 5) -> ()  [unwired: 1 out]
            }
          }
          frame Enabled {
          }
        }
      }
      frame "Dorsales" {
        n229 = Unbundle By Name(w604) -> ("Dorsales"=w602:i32)
        n230 = To Unsigned Byte Integer(number=w602) -> (unsigned 8bit integer=w603:u8)
        n231 = Build Array(w603) -> (w608:u8[])
        n232 = Byte Array To String(unsigned byte array=w608) -> (string=w606:string)
        n233 = Concatenate Strings("6", w606) -> (w605:string)
        n234 = String Length(string=w605) -> (length=w611:i32)
        n235 = for {
          N: w611 -> [_]
          tunnel: w614 -> [w653]
          tunnel: w615 -> [w652]
          tunnel: w605 -> [w649]
          tunnel: [w646] -> w609
          tunnel: [w645] -> w610
          i -> [w647]
          n236 = String Subset(string=w649, offset (0)=w647, length (rest)=1 ("length (rest)")) -> (substring=w650:string)
          n237 = VISA Write(VISA resource name=w652, write buffer=w650, error in (no error)=w653) -> (VISA resource name out=w645:refnum<visa-resource-name>, error out=w646:errorcluster)  [unwired: 1 out]
          n238 = Wait Until Next ms Multiple(millisecond multiple=u32 5) -> ()  [unwired: 1 out]
        }
        n239 = disable-structure shown="Disabled" {
          disable-tunnel: [w627 w643] -> w613
          disable-tunnel: [w626 w644] -> w612
          disable-tunnel: w610 -> [w621 w644]
          disable-tunnel: w609 -> [w617 w643]
          frame Disabled {
            n240 = call "Timer2.vi"("error in (no error)"=w617, "Reset"=TRUE) -> ("error out"=w616:errorcluster)  [unwired: 7 in, 2 out]
            n241 = while {
              tunnel: w621 -> [w633]
              tunnel: [w633] -> w620
              tunnel: [w631] -> w619
              tunnel: w616 -> [w632]
              stop <- w630 stop-if-true
              n242 = call "Timer2.vi"("error in (no error)"=w632, "Time Target (s)"=0.25, "Pause"=TRUE) -> ("error out"=w631:errorcluster, "Time has Elapsed"=w630:bool)  [unwired: 6 in, 1 out]
            }
            n243 = property class="Instr"(reference=w620, error in=w619) -> (reference out=w624:refnum<visa-resource-name>, error out=w623:errorcluster, "Bytes at Port"=w622:u32)
            n244 = for {
              N: w622 -> [_]
              tunnel: w623 -> [w641]
              tunnel: w624 -> [w640]
              shift-right: [w635] -> _
              shift-left: "" -> [w639]
              tunnel: [w638] -> w627
              tunnel: [w637] -> w626
              n245 = VISA Read(VISA resource name=w640, byte count=u32 1, error in (no error)=w641) -> (VISA resource name out=w637:refnum<visa-resource-name>, read buffer=w634:string, error out=w638:errorcluster)  [unwired: 1 out]
              n246 = Concatenate Strings(w639, w634) -> (w635:string)
              n247 = Wait Until Next ms Multiple(millisecond multiple=u32 5) -> ()  [unwired: 1 out]
            }
          }
          frame Enabled {
          }
        }
      }
      frame "Trapecio" {
        n248 = Unbundle By Name(w656) -> ("Trapecio"=w654:i32)
        n249 = To Unsigned Byte Integer(number=w654) -> (unsigned 8bit integer=w655:u8)
        n250 = Build Array(w655) -> (w660:u8[])
        n251 = Byte Array To String(unsigned byte array=w660) -> (string=w658:string)
        n252 = Concatenate Strings("7", w658) -> (w657:string)
        n253 = String Length(string=w657) -> (length=w663:i32)
        n254 = for {
          N: w663 -> [_]
          tunnel: w666 -> [w705]
          tunnel: w667 -> [w704]
          tunnel: w657 -> [w701]
          tunnel: [w698] -> w661
          tunnel: [w697] -> w662
          i -> [w699]
          n255 = String Subset(string=w701, offset (0)=w699, length (rest)=1 ("length (rest)")) -> (substring=w702:string)
          n256 = VISA Write(VISA resource name=w704, write buffer=w702, error in (no error)=w705) -> (VISA resource name out=w697:refnum<visa-resource-name>, error out=w698:errorcluster)  [unwired: 1 out]
          n257 = Wait Until Next ms Multiple(millisecond multiple=u32 5) -> ()  [unwired: 1 out]
        }
        n258 = disable-structure shown="Disabled" {
          disable-tunnel: [w679 w695] -> w665
          disable-tunnel: [w678 w696] -> w664
          disable-tunnel: w662 -> [w673 w696]
          disable-tunnel: w661 -> [w669 w695]
          frame Disabled {
            n259 = call "Timer2.vi"("error in (no error)"=w669, "Reset"=TRUE) -> ("error out"=w668:errorcluster)  [unwired: 7 in, 2 out]
            n260 = while {
              tunnel: w673 -> [w685]
              tunnel: [w685] -> w672
              tunnel: [w683] -> w671
              tunnel: w668 -> [w684]
              stop <- w682 stop-if-true
              n261 = call "Timer2.vi"("error in (no error)"=w684, "Time Target (s)"=0.25, "Pause"=TRUE) -> ("error out"=w683:errorcluster, "Time has Elapsed"=w682:bool)  [unwired: 6 in, 1 out]
            }
            n262 = property class="Instr"(reference=w672, error in=w671) -> (reference out=w676:refnum<visa-resource-name>, error out=w675:errorcluster, "Bytes at Port"=w674:u32)
            n263 = for {
              N: w674 -> [_]
              tunnel: w675 -> [w693]
              tunnel: w676 -> [w692]
              shift-right: [w687] -> _
              shift-left: "" -> [w691]
              tunnel: [w690] -> w679
              tunnel: [w689] -> w678
              n264 = VISA Read(VISA resource name=w692, byte count=u32 1, error in (no error)=w693) -> (VISA resource name out=w689:refnum<visa-resource-name>, read buffer=w686:string, error out=w690:errorcluster)  [unwired: 1 out]
              n265 = Concatenate Strings(w691, w686) -> (w687:string)
              n266 = Wait Until Next ms Multiple(millisecond multiple=u32 5) -> ()  [unwired: 1 out]
            }
          }
          frame Enabled {
          }
        }
      }
      frame "Pectorales" {
        n267 = Unbundle By Name(w708) -> ("Pectorales"=w706:i32)
        n268 = To Unsigned Byte Integer(number=w706) -> (unsigned 8bit integer=w707:u8)
        n269 = Build Array(w707) -> (w712:u8[])
        n270 = Byte Array To String(unsigned byte array=w712) -> (string=w710:string)
        n271 = Concatenate Strings("8", w710) -> (w709:string)
        n272 = String Length(string=w709) -> (length=w715:i32)
        n273 = for {
          N: w715 -> [_]
          tunnel: w718 -> [w757]
          tunnel: w719 -> [w756]
          tunnel: w709 -> [w753]
          tunnel: [w750] -> w713
          tunnel: [w749] -> w714
          i -> [w751]
          n274 = String Subset(string=w753, offset (0)=w751, length (rest)=1 ("length (rest)")) -> (substring=w754:string)
          n275 = VISA Write(VISA resource name=w756, write buffer=w754, error in (no error)=w757) -> (VISA resource name out=w749:refnum<visa-resource-name>, error out=w750:errorcluster)  [unwired: 1 out]
          n276 = Wait Until Next ms Multiple(millisecond multiple=u32 5) -> ()  [unwired: 1 out]
        }
        n277 = disable-structure shown="Disabled" {
          disable-tunnel: [w731 w747] -> w717
          disable-tunnel: [w730 w748] -> w716
          disable-tunnel: w714 -> [w725 w748]
          disable-tunnel: w713 -> [w721 w747]
          frame Disabled {
            n278 = call "Timer2.vi"("error in (no error)"=w721, "Reset"=TRUE) -> ("error out"=w720:errorcluster)  [unwired: 7 in, 2 out]
            n279 = while {
              tunnel: w725 -> [w737]
              tunnel: [w737] -> w724
              tunnel: [w735] -> w723
              tunnel: w720 -> [w736]
              stop <- w734 stop-if-true
              n280 = call "Timer2.vi"("error in (no error)"=w736, "Time Target (s)"=0.25, "Pause"=TRUE) -> ("error out"=w735:errorcluster, "Time has Elapsed"=w734:bool)  [unwired: 6 in, 1 out]
            }
            n281 = property class="Instr"(reference=w724, error in=w723) -> (reference out=w728:refnum<visa-resource-name>, error out=w727:errorcluster, "Bytes at Port"=w726:u32)
            n282 = for {
              N: w726 -> [_]
              tunnel: w727 -> [w745]
              tunnel: w728 -> [w744]
              shift-right: [w739] -> _
              shift-left: "" -> [w743]
              tunnel: [w742] -> w731
              tunnel: [w741] -> w730
              n283 = VISA Read(VISA resource name=w744, byte count=u32 1, error in (no error)=w745) -> (VISA resource name out=w741:refnum<visa-resource-name>, read buffer=w738:string, error out=w742:errorcluster)  [unwired: 1 out]
              n284 = Concatenate Strings(w743, w738) -> (w739:string)
              n285 = Wait Until Next ms Multiple(millisecond multiple=u32 5) -> ()  [unwired: 1 out]
            }
          }
          frame Enabled {
          }
        }
      }
      frame "Biceps" {
        n286 = Unbundle By Name(w760) -> ("Biceps"=w758:i32)
        n287 = To Unsigned Byte Integer(number=w758) -> (unsigned 8bit integer=w759:u8)
        n288 = Build Array(w759) -> (w764:u8[])
        n289 = Byte Array To String(unsigned byte array=w764) -> (string=w762:string)
        n290 = Concatenate Strings("9", w762) -> (w761:string)
        n291 = String Length(string=w761) -> (length=w767:i32)
        n292 = for {
          N: w767 -> [_]
          tunnel: w770 -> [w809]
          tunnel: w771 -> [w808]
          tunnel: w761 -> [w805]
          tunnel: [w802] -> w765
          tunnel: [w801] -> w766
          i -> [w803]
          n293 = String Subset(string=w805, offset (0)=w803, length (rest)=1 ("length (rest)")) -> (substring=w806:string)
          n294 = VISA Write(VISA resource name=w808, write buffer=w806, error in (no error)=w809) -> (VISA resource name out=w801:refnum<visa-resource-name>, error out=w802:errorcluster)  [unwired: 1 out]
          n295 = Wait Until Next ms Multiple(millisecond multiple=u32 5) -> ()  [unwired: 1 out]
        }
        n296 = disable-structure shown="Disabled" {
          disable-tunnel: [w783 w799] -> w769
          disable-tunnel: [w782 w800] -> w768
          disable-tunnel: w766 -> [w777 w800]
          disable-tunnel: w765 -> [w773 w799]
          frame Disabled {
            n297 = call "Timer2.vi"("error in (no error)"=w773, "Reset"=TRUE) -> ("error out"=w772:errorcluster)  [unwired: 7 in, 2 out]
            n298 = while {
              tunnel: w777 -> [w789]
              tunnel: [w789] -> w776
              tunnel: [w787] -> w775
              tunnel: w772 -> [w788]
              stop <- w786 stop-if-true
              n299 = call "Timer2.vi"("error in (no error)"=w788, "Time Target (s)"=0.25, "Pause"=TRUE) -> ("error out"=w787:errorcluster, "Time has Elapsed"=w786:bool)  [unwired: 6 in, 1 out]
            }
            n300 = property class="Instr"(reference=w776, error in=w775) -> (reference out=w780:refnum<visa-resource-name>, error out=w779:errorcluster, "Bytes at Port"=w778:u32)
            n301 = for {
              N: w778 -> [_]
              tunnel: w779 -> [w797]
              tunnel: w780 -> [w796]
              shift-right: [w791] -> _
              shift-left: "" -> [w795]
              tunnel: [w794] -> w783
              tunnel: [w793] -> w782
              n302 = VISA Read(VISA resource name=w796, byte count=u32 1, error in (no error)=w797) -> (VISA resource name out=w793:refnum<visa-resource-name>, read buffer=w790:string, error out=w794:errorcluster)  [unwired: 1 out]
              n303 = Concatenate Strings(w795, w790) -> (w791:string)
              n304 = Wait Until Next ms Multiple(millisecond multiple=u32 5) -> ()  [unwired: 1 out]
            }
          }
          frame Enabled {
          }
        }
      }
      frame "Opcional" {
        n305 = Unbundle By Name(w812) -> ("Opcional"=w810:i32)
        n306 = To Unsigned Byte Integer(number=w810) -> (unsigned 8bit integer=w811:u8)
        n307 = Build Array(w811) -> (w816:u8[])
        n308 = Byte Array To String(unsigned byte array=w816) -> (string=w814:string)
        n309 = Concatenate Strings("10", w814) -> (w813:string)
        n310 = String Length(string=w813) -> (length=w819:i32)
        n311 = for {
          N: w819 -> [_]
          tunnel: w822 -> [w861]
          tunnel: w823 -> [w860]
          tunnel: w813 -> [w857]
          tunnel: [w854] -> w817
          tunnel: [w853] -> w818
          i -> [w855]
          n312 = String Subset(string=w857, offset (0)=w855, length (rest)=1 ("length (rest)")) -> (substring=w858:string)
          n313 = VISA Write(VISA resource name=w860, write buffer=w858, error in (no error)=w861) -> (VISA resource name out=w853:refnum<visa-resource-name>, error out=w854:errorcluster)  [unwired: 1 out]
          n314 = Wait Until Next ms Multiple(millisecond multiple=u32 5) -> ()  [unwired: 1 out]
        }
        n315 = disable-structure shown="Disabled" {
          disable-tunnel: [w835 w851] -> w821
          disable-tunnel: [w834 w852] -> w820
          disable-tunnel: w818 -> [w829 w852]
          disable-tunnel: w817 -> [w825 w851]
          frame Disabled {
            n316 = call "Timer2.vi"("error in (no error)"=w825, "Reset"=TRUE) -> ("error out"=w824:errorcluster)  [unwired: 7 in, 2 out]
            n317 = while {
              tunnel: w829 -> [w841]
              tunnel: [w841] -> w828
              tunnel: [w839] -> w827
              tunnel: w824 -> [w840]
              stop <- w838 stop-if-true
              n318 = call "Timer2.vi"("error in (no error)"=w840, "Time Target (s)"=0.25, "Pause"=TRUE) -> ("error out"=w839:errorcluster, "Time has Elapsed"=w838:bool)  [unwired: 6 in, 1 out]
            }
            n319 = property class="Instr"(reference=w828, error in=w827) -> (reference out=w832:refnum<visa-resource-name>, error out=w831:errorcluster, "Bytes at Port"=w830:u32)
            n320 = for {
              N: w830 -> [_]
              tunnel: w831 -> [w849]
              tunnel: w832 -> [w848]
              shift-right: [w843] -> _
              shift-left: "" -> [w847]
              tunnel: [w846] -> w835
              tunnel: [w845] -> w834
              n321 = VISA Read(VISA resource name=w848, byte count=u32 1, error in (no error)=w849) -> (VISA resource name out=w845:refnum<visa-resource-name>, read buffer=w842:string, error out=w846:errorcluster)  [unwired: 1 out]
              n322 = Concatenate Strings(w847, w842) -> (w843:string)
              n323 = Wait Until Next ms Multiple(millisecond multiple=u32 5) -> ()  [unwired: 1 out]
            }
          }
          frame Enabled {
          }
        }
      }
    }
    n324 = local read "Stop"() -> (w70:bool)
    n325 = local read "Back"() -> (w71:bool)
    n326 = Or(x=w70, y=w71) -> (x .or. y?=w69:bool)
  }
  n327 = while {
    tunnel: w12 -> [_]
    tunnel: w4 -> [w866]
    shift-right: [w864] -> _
    shift-left: w5 -> [w865]
    shift-right: [w862] -> w1
    shift-left: w2 -> [w863]
    stop <- w868 stop-if-true
    n328 = event shown="[11] \"Add Button\": Value Change" {
      selector: _ -> [_ _ _ _ _ _ _ _ _ _ _ _ _ _ _ _ _ _ _ _ _]
      dyn-events: _ -> [_ _ _ _ _ _ _ _ _ _ _ _ _ _ _ _ _ _ _ _ _]
      timeout: 300 -> [_ _ _ _ _ _ _ _ _ _ _ _ _ _ _ _ _ _ _ _ _]
      tunnel: [_ FALSE FALSE FALSE FALSE FALSE FALSE FALSE FALSE FALSE FALSE _ _ _ "Stop" TRUE ("Stop") FALSE ("Stop") FALSE ("Stop") FALSE ("Stop") FALSE ("Stop") FALSE ("Stop")] -> w868
      tunnel: w866 -> [w872 _ _ _ _ _ _ _ _ _ _ w1110 w1260 w1375 _ _ _ _ w1494 w1547 _]
      tunnel: w865 -> [w871 w970 w984 w999 w1013 w1027 w1041 w1055 w1069 w1083 w1097 w1113 w1262 w1379 w1448 w1452 w1463 w1479 w1496 w1548 w1553]
      tunnel: [w870 w971 w985 w998 w1012 w1026 w1040 w1054 w1068 w1082 w1096 w1114 w1263 w1380 w1448 w1450 w1461 w1479 w1482 w1499 w1552] -> w864
      tunnel: w863 -> [w873 _ _ _ _ _ _ _ _ _ _ w1111 w1259 w1376 _ _ _ _ w1493 w1546 _]
      tunnel: [w869 _ _ _ _ _ _ _ _ _ _ _ _ _ _ _ _ _ _ _ _] -> w862
      event Timeout {
        n329 = event-data() -> ()  [unwired: 1 in, 3 out]
        n330 = Unbundle By Name(w871) -> ("Label"=w890:string, "Cuadriceps"=w889:i32, "Isquiotibiales"=w888:i32, "Gluteos"=w887:i32, "Abdomen"=w886:i32, "Lumbares"=w885:i32, "Dorsales"=w884:i32, "Trapecio"=w883:i32, "Pectorales"=w882:i32, "Biceps"=w881:i32, "Opcional"=w880:i32)
        n331 = Unbundle By Name(w871) -> ("Impulso"=w878:i32, "Tiempo"=w877:i32)
        n332 = Unbundle By Name(w871) -> ("Label"=w876:string, "Impulso"=w875:i32, "Ruptura"=w874:i32)
        n333 = local read "Boolean"() -> (w891:bool)
        n334 = case shown="\"Inicio\", Default" w890 {
          selector: w890 -> [w922 w927 w932 w937 w942 w947 w952 w957 w962 w967 w969]
          tunnel: [w922 w927 w932 w937 w942 w947 w952 w957 w962 w967 w969] -> _
          tunnel: [w918 w923 w928 w933 w938 w943 w948 w953 w958 w963 0] -> w879
          tunnel: w889 -> [w918 _ _ _ _ _ _ _ _ _ _]
          tunnel: w888 -> [_ w923 _ _ _ _ _ _ _ _ _]
          tunnel: w887 -> [_ _ w928 _ _ _ _ _ _ _ _]
          tunnel: w886 -> [_ _ _ w933 _ _ _ _ _ _ _]
          tunnel: w885 -> [_ _ _ _ w938 _ _ _ _ _ _]
          tunnel: w884 -> [_ _ _ _ _ w943 _ _ _ _ _]
          tunnel: w883 -> [_ _ _ _ _ _ w948 _ _ _ _]
          tunnel: w882 -> [_ _ _ _ _ _ _ w953 _ _ _]
          tunnel: w881 -> [_ _ _ _ _ _ _ _ w958 _ _]
          tunnel: w880 -> [_ _ _ _ _ _ _ _ _ w963 _]
          frame "Cuadriceps" {
            n335 = Number To Decimal String(number=w918) -> (decimal integer string=w921:string)  [unwired: 1 in]
            n336 = Concatenate Strings(w921, "%" ("string")) -> (→"Cuadríceps %":string)
          }
          frame "Isquiotibiales" {
            n337 = Number To Decimal String(number=w923) -> (decimal integer string=w926:string)  [unwired: 1 in]
            n338 = Concatenate Strings(w926, "%" ("string")) -> (→"Isquiotibiales %":string)
          }
          frame "Gluteos" {
            n339 = Number To Decimal String(number=w928) -> (decimal integer string=w931:string)  [unwired: 1 in]
            n340 = Concatenate Strings(w931, "%" ("string")) -> (→"Gluteos %":string)
          }
          frame "Abdomen" {
            n341 = Number To Decimal String(number=w933) -> (decimal integer string=w936:string)  [unwired: 1 in]
            n342 = Concatenate Strings(w936, "%" ("string")) -> (→"Abdomen %":string)
          }
          frame "Lumbares" {
            n343 = Number To Decimal String(number=w938) -> (decimal integer string=w941:string)  [unwired: 1 in]
            n344 = Concatenate Strings(w941, "%" ("string")) -> (→"Lumbares %":string)
          }
          frame "Dorsales" {
            n345 = Number To Decimal String(number=w943) -> (decimal integer string=w946:string)  [unwired: 1 in]
            n346 = Concatenate Strings(w946, "%" ("string")) -> (→"Dorsales %":string)
          }
          frame "Trapecio" {
            n347 = Number To Decimal String(number=w948) -> (decimal integer string=w951:string)  [unwired: 1 in]
            n348 = Concatenate Strings(w951, "%" ("string")) -> (→"Trapecio %":string)
          }
          frame "Pectorales" {
            n349 = Number To Decimal String(number=w953) -> (decimal integer string=w956:string)  [unwired: 1 in]
            n350 = Concatenate Strings(w956, "%" ("string")) -> (→"Pectorales %":string)
          }
          frame "Biceps" {
            n351 = Number To Decimal String(number=w958) -> (decimal integer string=w961:string)  [unwired: 1 in]
            n352 = Concatenate Strings(w961, "%" ("string")) -> (→"Biceps %":string)
          }
          frame "Opcional" {
            n353 = Number To Decimal String(number=w963) -> (decimal integer string=w966:string)  [unwired: 1 in]
            n354 = Concatenate Strings(w966, "%" ("string")) -> (→"Opcional %":string)
          }
          frame "Inicio", Default {
          }
        }
        "Horizontal Graduated Bar" <- w879
        n355 = case shown="True" w891 {
          tunnel: w877 -> [_ w905]
          tunnel: w878 -> [_ w904]
          frame False {
            n356 = property on="Start" class="Bool (strict)"("BoolText.Text"="Start / Inicio" ("Boolean Text.Text")) -> ()  [unwired: 2 in, 2 out]
          }
          frame True {
            n357 = Number To Decimal String(number=w904) -> (decimal integer string=→"Impulso":string)  [unwired: 1 in]
            n358 = Multiply(x=w905, y=60) -> (x*y=w908:i32)
            n359 = property on="Start" class="Bool (strict)"("BoolText.Text"="Stop / Parar" ("Boolean Text.Text")) -> ()  [unwired: 2 in, 2 out]
            n360 = call "Elapsed Time"("Time Target (s)"=w908) -> ("Elapsed Time (s)"=w914:dbl)  [unwired: 11 in, 7 out]
            n361 = Subtract(x=w908, y=w914) -> (x-y=w913:dbl)
            n362 = To Time Stamp(1:w914) -> (0:w915:timestamp)
            n363 = To Time Stamp(1:w913) -> (0:w910:timestamp)
            n364 = Format Date/Time String(time format string (%c)="%M : %S", seconds (now)=w915) -> (date/time string=→"Tiempo Transcurrido":string)  [unwired: 1 in]
            n365 = Format Date/Time String(time format string (%c)="%M : %S", seconds (now)=w910) -> (date/time string=→"Tiempo Restante":string)  [unwired: 1 in]
          }
        }
        n366 = local write "Slider"(w879) -> ()
        n367 = case shown="\"Start\"" w876 {
          tunnel: w875 -> [_ w902]
          tunnel: w874 -> [_ w896]
          tunnel: w873 -> [w893 w898]
          tunnel: w872 -> [_ w899]
          tunnel: w871 -> [w894 w900]
          tunnel: [w894 w897] -> w870
          tunnel: [w893 w895] -> w869
          frame "Inicio", Default {
          }
          frame "Start" {
            n368 = Bundle By Name(cluster=w900, "Label"="Encender", "Impulso"=w902, "Ruptura"=w896) -> (w897:T1)
            n369 = Enqueue Element(queue=w899, element=w897, error in (no error)=w898) -> (error out=w895:errorcluster)  [unwired: 1 in, 2 out]
          }
        }
        n370 = Format Date/Time String() -> (date/time string=→"date/time string":string)  [unwired: 3 in]
      }
      event "Cuadriceps Bool": Value Change {
        n371 = event-data() -> ()  [unwired: 1 in, 6 out]
        n372 = Bundle By Name(cluster=cluster{"Color Box":u32, "Color Box 2":u32} {"Color Box"=12369084, "Color Box 2"=12369084}, "Color Box"=u32 16711680 ("Color Box 2")) -> (w980:cluster{"Color Box":u32, "Color Box 2":u32})
        n373 = Bundle By Name(cluster=cluster{"Color Box":u32, "Color Box 2":u32} {"Color Box"=12369084, "Color Box 2"=12369084}, "Color Box"=u32 12369084 ("Color Box 2")) -> (w975:cluster{"Color Box":u32, "Color Box 2":u32})
        n374 = Bundle By Name(cluster=w970, "Label"="Cuadriceps" ("Message")) -> (w971:T1)
        n375 = Insert Into Array(array=cluster{u32, u32}[] [] ("Colors [4]"), new element=w980) -> (w979:cluster{u32, u32}[])  [unwired: 1 in]
        n376 = Insert Into Array(array=cluster{u32, u32}[] [] ("Colors [4]"), new element=w975) -> (w973:cluster{u32, u32}[])  [unwired: 1 in]
        n377 = property on="Cuadriceps Bool" class="Bool"("Colors [4]"=w979) -> ()  [unwired: 2 in, 2 out]
        n378 = property on="Abdomen Bool" class="Bool"("Colors [4]"=w973) -> ()  [unwired: 2 in, 2 out]
        n379 = property on="Lumbares Bool" class="Bool"("Colors [4]"=w973) -> ()  [unwired: 2 in, 2 out]
        n380 = property on="Gluteos Bool" class="Bool"("Colors [4]"=w973) -> ()  [unwired: 2 in, 2 out]
        n381 = property on="Isquiotibiales Bool" class="Bool"("Colors [4]"=w973) -> ()  [unwired: 2 in, 2 out]
        n382 = property on="Pectorales Bool" class="Bool"("Colors [4]"=w973) -> ()  [unwired: 2 in, 2 out]
        n383 = property on="Dorsales Bool" class="Bool"("Colors [4]"=w973) -> ()  [unwired: 2 in, 2 out]
        n384 = property on="Trapecio Bool" class="Bool"("Colors [4]"=w973) -> ()  [unwired: 2 in, 2 out]
        n385 = property on="Opcional Bool" class="Bool"("Colors [4]"=w973) -> ()  [unwired: 2 in, 2 out]
        n386 = property on="Biceps Bool" class="Bool"("Colors [4]"=w973) -> ()  [unwired: 2 in, 2 out]
      }
      event "Isquiotibiales Bool": Value Change {
        n387 = event-data() -> ()  [unwired: 1 in, 6 out]
        n388 = Bundle By Name(cluster=cluster{"Color Box":u32, "Color Box 2":u32} {"Color Box"=12369084, "Color Box 2"=12369084}, "Color Box"=u32 16711680 ("Color Box 2")) -> (w994:cluster{"Color Box":u32, "Color Box 2":u32})
        n389 = Bundle By Name(cluster=cluster{"Color Box":u32, "Color Box 2":u32} {"Color Box"=12369084, "Color Box 2"=12369084}, "Color Box"=u32 12369084 ("Color Box 2")) -> (w990:cluster{"Color Box":u32, "Color Box 2":u32})
        n390 = Bundle By Name(cluster=w984, "Label"="Isquiotibiales" ("Message")) -> (w985:T1)
        n391 = Insert Into Array(array=cluster{u32, u32}[] [] ("Colors [4]"), new element=w994) -> (w988:cluster{u32, u32}[])  [unwired: 1 in]
        n392 = Insert Into Array(array=cluster{u32, u32}[] [] ("Colors [4]"), new element=w990) -> (w987:cluster{u32, u32}[])  [unwired: 1 in]
        n393 = property on="Isquiotibiales Bool" class="Bool"("Colors [4]"=w988) -> ()  [unwired: 2 in, 2 out]
        n394 = property on="Abdomen Bool" class="Bool"("Colors [4]"=w987) -> ()  [unwired: 2 in, 2 out]
        n395 = property on="Lumbares Bool" class="Bool"("Colors [4]"=w987) -> ()  [unwired: 2 in, 2 out]
        n396 = property on="Gluteos Bool" class="Bool"("Colors [4]"=w987) -> ()  [unwired: 2 in, 2 out]
        n397 = property on="Cuadriceps Bool" class="Bool"("Colors [4]"=w987) -> ()  [unwired: 2 in, 2 out]
        n398 = property on="Pectorales Bool" class="Bool"("Colors [4]"=w987) -> ()  [unwired: 2 in, 2 out]
        n399 = property on="Dorsales Bool" class="Bool"("Colors [4]"=w987) -> ()  [unwired: 2 in, 2 out]
        n400 = property on="Trapecio Bool" class="Bool"("Colors [4]"=w987) -> ()  [unwired: 2 in, 2 out]
        n401 = property on="Opcional Bool" class="Bool"("Colors [4]"=w987) -> ()  [unwired: 2 in, 2 out]
        n402 = property on="Biceps Bool" class="Bool"("Colors [4]"=w987) -> ()  [unwired: 2 in, 2 out]
      }
      event "Gluteos Bool": Value Change {
        n403 = event-data() -> ()  [unwired: 1 in, 6 out]
        n404 = Bundle By Name(cluster=cluster{"Color Box":u32, "Color Box 2":u32} {"Color Box"=12369084, "Color Box 2"=12369084}, "Color Box"=u32 16711680 ("Color Box 2")) -> (w1008:cluster{"Color Box":u32, "Color Box 2":u32})
        n405 = Bundle By Name(cluster=cluster{"Color Box":u32, "Color Box 2":u32} {"Color Box"=12369084, "Color Box 2"=12369084}, "Color Box"=u32 12369084 ("Color Box 2")) -> (w1004:cluster{"Color Box":u32, "Color Box 2":u32})
        n406 = Bundle By Name(cluster=w999, "Label"="Gluteos" ("Message")) -> (w998:T1)
        n407 = Insert Into Array(array=cluster{u32, u32}[] [] ("Colors [4]"), new element=w1008) -> (w1002:cluster{u32, u32}[])  [unwired: 1 in]
        n408 = Insert Into Array(array=cluster{u32, u32}[] [] ("Colors [4]"), new element=w1004) -> (w1001:cluster{u32, u32}[])  [unwired: 1 in]
        n409 = property on="Gluteos Bool" class="Bool"("Colors [4]"=w1002) -> ()  [unwired: 2 in, 2 out]
        n410 = property on="Abdomen Bool" class="Bool"("Colors [4]"=w1001) -> ()  [unwired: 2 in, 2 out]
        n411 = property on="Lumbares Bool" class="Bool"("Colors [4]"=w1001) -> ()  [unwired: 2 in, 2 out]
        n412 = property on="Isquiotibiales Bool" class="Bool"("Colors [4]"=w1001) -> ()  [unwired: 2 in, 2 out]
        n413 = property on="Cuadriceps Bool" class="Bool"("Colors [4]"=w1001) -> ()  [unwired: 2 in, 2 out]
        n414 = property on="Pectorales Bool" class="Bool"("Colors [4]"=w1001) -> ()  [unwired: 2 in, 2 out]
        n415 = property on="Dorsales Bool" class="Bool"("Colors [4]"=w1001) -> ()  [unwired: 2 in, 2 out]
        n416 = property on="Trapecio Bool" class="Bool"("Colors [4]"=w1001) -> ()  [unwired: 2 in, 2 out]
        n417 = property on="Opcional Bool" class="Bool"("Colors [4]"=w1001) -> ()  [unwired: 2 in, 2 out]
        n418 = property on="Biceps Bool" class="Bool"("Colors [4]"=w1001) -> ()  [unwired: 2 in, 2 out]
      }
      event "Abdomen Bool": Value Change {
        n419 = event-data() -> ()  [unwired: 1 in, 6 out]
        n420 = Bundle By Name(cluster=cluster{"Color Box":u32, "Color Box 2":u32} {"Color Box"=12369084, "Color Box 2"=12369084}, "Color Box"=u32 16711680 ("Color Box 2")) -> (w1022:cluster{"Color Box":u32, "Color Box 2":u32})
        n421 = Bundle By Name(cluster=cluster{"Color Box":u32, "Color Box 2":u32} {"Color Box"=12369084, "Color Box 2"=12369084}, "Color Box"=u32 12369084 ("Color Box 2")) -> (w1018:cluster{"Color Box":u32, "Color Box 2":u32})
        n422 = Bundle By Name(cluster=w1013, "Label"="Abdomen" ("Message")) -> (w1012:T1)
        n423 = Insert Into Array(array=cluster{u32, u32}[] [] ("Colors [4]"), new element=w1022) -> (w1016:cluster{u32, u32}[])  [unwired: 1 in]
        n424 = Insert Into Array(array=cluster{u32, u32}[] [] ("Colors [4]"), new element=w1018) -> (w1015:cluster{u32, u32}[])  [unwired: 1 in]
        n425 = property on="Abdomen Bool" class="Bool"("Colors [4]"=w1016) -> ()  [unwired: 2 in, 2 out]
        n426 = property on="Gluteos Bool" class="Bool"("Colors [4]"=w1015) -> ()  [unwired: 2 in, 2 out]
        n427 = property on="Lumbares Bool" class="Bool"("Colors [4]"=w1015) -> ()  [unwired: 2 in, 2 out]
        n428 = property on="Isquiotibiales Bool" class="Bool"("Colors [4]"=w1015) -> ()  [unwired: 2 in, 2 out]
        n429 = property on="Cuadriceps Bool" class="Bool"("Colors [4]"=w1015) -> ()  [unwired: 2 in, 2 out]
        n430 = property on="Pectorales Bool" class="Bool"("Colors [4]"=w1015) -> ()  [unwired: 2 in, 2 out]
        n431 = property on="Dorsales Bool" class="Bool"("Colors [4]"=w1015) -> ()  [unwired: 2 in, 2 out]
        n432 = property on="Trapecio Bool" class="Bool"("Colors [4]"=w1015) -> ()  [unwired: 2 in, 2 out]
        n433 = property on="Opcional Bool" class="Bool"("Colors [4]"=w1015) -> ()  [unwired: 2 in, 2 out]
        n434 = property on="Biceps Bool" class="Bool"("Colors [4]"=w1015) -> ()  [unwired: 2 in, 2 out]
      }
      event "Lumbares Bool": Value Change {
        n435 = event-data() -> ()  [unwired: 1 in, 6 out]
        n436 = Bundle By Name(cluster=cluster{"Color Box":u32, "Color Box 2":u32} {"Color Box"=12369084, "Color Box 2"=12369084}, "Color Box"=u32 16711680 ("Color Box 2")) -> (w1036:cluster{"Color Box":u32, "Color Box 2":u32})
        n437 = Bundle By Name(cluster=cluster{"Color Box":u32, "Color Box 2":u32} {"Color Box"=12369084, "Color Box 2"=12369084}, "Color Box"=u32 12369084 ("Color Box 2")) -> (w1032:cluster{"Color Box":u32, "Color Box 2":u32})
        n438 = Insert Into Array(array=cluster{u32, u32}[] [] ("Colors [4]"), new element=w1036) -> (w1030:cluster{u32, u32}[])  [unwired: 1 in]
        n439 = Insert Into Array(array=cluster{u32, u32}[] [] ("Colors [4]"), new element=w1032) -> (w1029:cluster{u32, u32}[])  [unwired: 1 in]
        n440 = Bundle By Name(cluster=w1027, "Label"="Lumbares" ("Message")) -> (w1026:T1)
        n441 = property on="Lumbares Bool" class="Bool"("Colors [4]"=w1030) -> ()  [unwired: 2 in, 2 out]
        n442 = property on="Gluteos Bool" class="Bool"("Colors [4]"=w1029) -> ()  [unwired: 2 in, 2 out]
        n443 = property on="Abdomen Bool" class="Bool"("Colors [4]"=w1029) -> ()  [unwired: 2 in, 2 out]
        n444 = property on="Isquiotibiales Bool" class="Bool"("Colors [4]"=w1029) -> ()  [unwired: 2 in, 2 out]
        n445 = property on="Cuadriceps Bool" class="Bool"("Colors [4]"=w1029) -> ()  [unwired: 2 in, 2 out]
        n446 = property on="Pectorales Bool" class="Bool"("Colors [4]"=w1029) -> ()  [unwired: 2 in, 2 out]
        n447 = property on="Dorsales Bool" class="Bool"("Colors [4]"=w1029) -> ()  [unwired: 2 in, 2 out]
        n448 = property on="Trapecio Bool" class="Bool"("Colors [4]"=w1029) -> ()  [unwired: 2 in, 2 out]
        n449 = property on="Opcional Bool" class="Bool"("Colors [4]"=w1029) -> ()  [unwired: 2 in, 2 out]
        n450 = property on="Biceps Bool" class="Bool"("Colors [4]"=w1029) -> ()  [unwired: 2 in, 2 out]
      }
      event "Dorsales Bool": Value Change {
        n451 = event-data() -> ()  [unwired: 1 in, 6 out]
        n452 = Bundle By Name(cluster=cluster{"Color Box":u32, "Color Box 2":u32} {"Color Box"=12369084, "Color Box 2"=12369084}, "Color Box"=u32 16711680 ("Color Box 2")) -> (w1050:cluster{"Color Box":u32, "Color Box 2":u32})
        n453 = Bundle By Name(cluster=cluster{"Color Box":u32, "Color Box 2":u32} {"Color Box"=12369084, "Color Box 2"=12369084}, "Color Box"=u32 12369084 ("Color Box 2")) -> (w1046:cluster{"Color Box":u32, "Color Box 2":u32})
        n454 = Bundle By Name(cluster=w1041, "Label"="Dorsales" ("Message")) -> (w1040:T1)
        n455 = Insert Into Array(array=cluster{u32, u32}[] [] ("Colors [4]"), new element=w1050) -> (w1043:cluster{u32, u32}[])  [unwired: 1 in]
        n456 = Insert Into Array(array=cluster{u32, u32}[] [] ("Colors [4]"), new element=w1046) -> (w1044:cluster{u32, u32}[])  [unwired: 1 in]
        n457 = property on="Gluteos Bool" class="Bool"("Colors [4]"=w1044) -> ()  [unwired: 2 in, 2 out]
        n458 = property on="Abdomen Bool" class="Bool"("Colors [4]"=w1044) -> ()  [unwired: 2 in, 2 out]
        n459 = property on="Isquiotibiales Bool" class="Bool"("Colors [4]"=w1044) -> ()  [unwired: 2 in, 2 out]
        n460 = property on="Cuadriceps Bool" class="Bool"("Colors [4]"=w1044) -> ()  [unwired: 2 in, 2 out]
        n461 = property on="Dorsales Bool" class="Bool"("Colors [4]"=w1043) -> ()  [unwired: 2 in, 2 out]
        n462 = property on="Pectorales Bool" class="Bool"("Colors [4]"=w1044) -> ()  [unwired: 2 in, 2 out]
        n463 = property on="Lumbares Bool" class="Bool"("Colors [4]"=w1044) -> ()  [unwired: 2 in, 2 out]
        n464 = property on="Trapecio Bool" class="Bool"("Colors [4]"=w1044) -> ()  [unwired: 2 in, 2 out]
        n465 = property on="Opcional Bool" class="Bool"("Colors [4]"=w1044) -> ()  [unwired: 2 in, 2 out]
        n466 = property on="Biceps Bool" class="Bool"("Colors [4]"=w1044) -> ()  [unwired: 2 in, 2 out]
      }
      event "Trapecio Bool": Value Change {
        n467 = event-data() -> ()  [unwired: 1 in, 6 out]
        n468 = Bundle By Name(cluster=cluster{"Color Box":u32, "Color Box 2":u32} {"Color Box"=12369084, "Color Box 2"=12369084}, "Color Box"=u32 16711680 ("Color Box 2")) -> (w1064:cluster{"Color Box":u32, "Color Box 2":u32})
        n469 = Bundle By Name(cluster=cluster{"Color Box":u32, "Color Box 2":u32} {"Color Box"=12369084, "Color Box 2"=12369084}, "Color Box"=u32 12369084 ("Color Box 2")) -> (w1060:cluster{"Color Box":u32, "Color Box 2":u32})
        n470 = Bundle By Name(cluster=w1055, "Label"="Trapecio" ("Message")) -> (w1054:T1)
        n471 = Insert Into Array(array=cluster{u32, u32}[] [] ("Colors [4]"), new element=w1064) -> (w1057:cluster{u32, u32}[])  [unwired: 1 in]
        n472 = Insert Into Array(array=cluster{u32, u32}[] [] ("Colors [4]"), new element=w1060) -> (w1058:cluster{u32, u32}[])  [unwired: 1 in]
        n473 = property on="Trapecio Bool" class="Bool"("Colors [4]"=w1057) -> ()  [unwired: 2 in, 2 out]
        n474 = property on="Gluteos Bool" class="Bool"("Colors [4]"=w1058) -> ()  [unwired: 2 in, 2 out]
        n475 = property on="Abdomen Bool" class="Bool"("Colors [4]"=w1058) -> ()  [unwired: 2 in, 2 out]
        n476 = property on="Isquiotibiales Bool" class="Bool"("Colors [4]"=w1058) -> ()  [unwired: 2 in, 2 out]
        n477 = property on="Cuadriceps Bool" class="Bool"("Colors [4]"=w1058) -> ()  [unwired: 2 in, 2 out]
        n478 = property on="Pectorales Bool" class="Bool"("Colors [4]"=w1058) -> ()  [unwired: 2 in, 2 out]
        n479 = property on="Lumbares Bool" class="Bool"("Colors [4]"=w1058) -> ()  [unwired: 2 in, 2 out]
        n480 = property on="Dorsales Bool" class="Bool"("Colors [4]"=w1058) -> ()  [unwired: 2 in, 2 out]
        n481 = property on="Opcional Bool" class="Bool"("Colors [4]"=w1058) -> ()  [unwired: 2 in, 2 out]
        n482 = property on="Biceps Bool" class="Bool"("Colors [4]"=w1058) -> ()  [unwired: 2 in, 2 out]
      }
      event "Pectorales Bool": Value Change {
        n483 = event-data() -> ()  [unwired: 1 in, 6 out]
        n484 = Bundle By Name(cluster=cluster{"Color Box":u32, "Color Box 2":u32} {"Color Box"=12369084, "Color Box 2"=12369084}, "Color Box"=u32 16711680 ("Color Box 2")) -> (w1078:cluster{"Color Box":u32, "Color Box 2":u32})
        n485 = Bundle By Name(cluster=cluster{"Color Box":u32, "Color Box 2":u32} {"Color Box"=12369084, "Color Box 2"=12369084}, "Color Box"=u32 12369084 ("Color Box 2")) -> (w1074:cluster{"Color Box":u32, "Color Box 2":u32})
        n486 = Bundle By Name(cluster=w1069, "Label"="Pectorales" ("Message")) -> (w1068:T1)
        n487 = Insert Into Array(array=cluster{u32, u32}[] [] ("Colors [4]"), new element=w1078) -> (w1071:cluster{u32, u32}[])  [unwired: 1 in]
        n488 = Insert Into Array(array=cluster{u32, u32}[] [] ("Colors [4]"), new element=w1074) -> (w1072:cluster{u32, u32}[])  [unwired: 1 in]
        n489 = property on="Pectorales Bool" class="Bool"("Colors [4]"=w1071) -> ()  [unwired: 2 in, 2 out]
        n490 = property on="Gluteos Bool" class="Bool"("Colors [4]"=w1072) -> ()  [unwired: 2 in, 2 out]
        n491 = property on="Abdomen Bool" class="Bool"("Colors [4]"=w1072) -> ()  [unwired: 2 in, 2 out]
        n492 = property on="Isquiotibiales Bool" class="Bool"("Colors [4]"=w1072) -> ()  [unwired: 2 in, 2 out]
        n493 = property on="Cuadriceps Bool" class="Bool"("Colors [4]"=w1072) -> ()  [unwired: 2 in, 2 out]
        n494 = property on="Trapecio Bool" class="Bool"("Colors [4]"=w1072) -> ()  [unwired: 2 in, 2 out]
        n495 = property on="Lumbares Bool" class="Bool"("Colors [4]"=w1072) -> ()  [unwired: 2 in, 2 out]
        n496 = property on="Dorsales Bool" class="Bool"("Colors [4]"=w1072) -> ()  [unwired: 2 in, 2 out]
        n497 = property on="Opcional Bool" class="Bool"("Colors [4]"=w1072) -> ()  [unwired: 2 in, 2 out]
        n498 = property on="Biceps Bool" class="Bool"("Colors [4]"=w1072) -> ()  [unwired: 2 in, 2 out]
      }
      event "Biceps Bool": Value Change {
        n499 = event-data() -> ()  [unwired: 1 in, 6 out]
        n500 = Bundle By Name(cluster=cluster{"Color Box":u32, "Color Box 2":u32} {"Color Box"=12369084, "Color Box 2"=12369084}, "Color Box"=u32 16711680 ("Color Box 2")) -> (w1092:cluster{"Color Box":u32, "Color Box 2":u32})
        n501 = Bundle By Name(cluster=cluster{"Color Box":u32, "Color Box 2":u32} {"Color Box"=12369084, "Color Box 2"=12369084}, "Color Box"=u32 12369084 ("Color Box 2")) -> (w1088:cluster{"Color Box":u32, "Color Box 2":u32})
        n502 = Bundle By Name(cluster=w1083, "Label"="Biceps" ("Message")) -> (w1082:T1)
        n503 = Insert Into Array(array=cluster{u32, u32}[] [] ("Colors [4]"), new element=w1092) -> (w1085:cluster{u32, u32}[])  [unwired: 1 in]
        n504 = Insert Into Array(array=cluster{u32, u32}[] [] ("Colors [4]"), new element=w1088) -> (w1086:cluster{u32, u32}[])  [unwired: 1 in]
        n505 = property on="Biceps Bool" class="Bool"("Colors [4]"=w1085) -> ()  [unwired: 2 in, 2 out]
        n506 = property on="Gluteos Bool" class="Bool"("Colors [4]"=w1086) -> ()  [unwired: 2 in, 2 out]
        n507 = property on="Abdomen Bool" class="Bool"("Colors [4]"=w1086) -> ()  [unwired: 2 in, 2 out]
        n508 = property on="Isquiotibiales Bool" class="Bool"("Colors [4]"=w1086) -> ()  [unwired: 2 in, 2 out]
        n509 = property on="Cuadriceps Bool" class="Bool"("Colors [4]"=w1086) -> ()  [unwired: 2 in, 2 out]
        n510 = property on="Trapecio Bool" class="Bool"("Colors [4]"=w1086) -> ()  [unwired: 2 in, 2 out]
        n511 = property on="Lumbares Bool" class="Bool"("Colors [4]"=w1086) -> ()  [unwired: 2 in, 2 out]
        n512 = property on="Dorsales Bool" class="Bool"("Colors [4]"=w1086) -> ()  [unwired: 2 in, 2 out]
        n513 = property on="Opcional Bool" class="Bool"("Colors [4]"=w1086) -> ()  [unwired: 2 in, 2 out]
        n514 = property on="Pectorales Bool" class="Bool"("Colors [4]"=w1086) -> ()  [unwired: 2 in, 2 out]
      }
      event "Opcional Bool": Value Change {
        n515 = event-data() -> ()  [unwired: 1 in, 6 out]
        n516 = Bundle By Name(cluster=cluster{"Color Box":u32, "Color Box 2":u32} {"Color Box"=12369084, "Color Box 2"=12369084}, "Color Box"=u32 16711680 ("Color Box 2")) -> (w1106:cluster{"Color Box":u32, "Color Box 2":u32})
        n517 = Bundle By Name(cluster=cluster{"Color Box":u32, "Color Box 2":u32} {"Color Box"=12369084, "Color Box 2"=12369084}, "Color Box"=u32 12369084 ("Color Box 2")) -> (w1102:cluster{"Color Box":u32, "Color Box 2":u32})
        n518 = Bundle By Name(cluster=w1097, "Label"="Opcional" ("Message")) -> (w1096:T1)
        n519 = Insert Into Array(array=cluster{u32, u32}[] [] ("Colors [4]"), new element=w1106) -> (w1099:cluster{u32, u32}[])  [unwired: 1 in]
        n520 = Insert Into Array(array=cluster{u32, u32}[] [] ("Colors [4]"), new element=w1102) -> (w1100:cluster{u32, u32}[])  [unwired: 1 in]
        n521 = property on="Opcional Bool" class="Bool"("Colors [4]"=w1099) -> ()  [unwired: 2 in, 2 out]
        n522 = property on="Gluteos Bool" class="Bool"("Colors [4]"=w1100) -> ()  [unwired: 2 in, 2 out]
        n523 = property on="Abdomen Bool" class="Bool"("Colors [4]"=w1100) -> ()  [unwired: 2 in, 2 out]
        n524 = property on="Isquiotibiales Bool" class="Bool"("Colors [4]"=w1100) -> ()  [unwired: 2 in, 2 out]
        n525 = property on="Cuadriceps Bool" class="Bool"("Colors [4]"=w1100) -> ()  [unwired: 2 in, 2 out]
        n526 = property on="Trapecio Bool" class="Bool"("Colors [4]"=w1100) -> ()  [unwired: 2 in, 2 out]
        n527 = property on="Lumbares Bool" class="Bool"("Colors [4]"=w1100) -> ()  [unwired: 2 in, 2 out]
        n528 = property on="Dorsales Bool" class="Bool"("Colors [4]"=w1100) -> ()  [unwired: 2 in, 2 out]
        n529 = property on="Biceps Bool" class="Bool"("Colors [4]"=w1100) -> ()  [unwired: 2 in, 2 out]
        n530 = property on="Pectorales Bool" class="Bool"("Colors [4]"=w1100) -> ()  [unwired: 2 in, 2 out]
      }
      event "Add Button": Value Change {
        n531 = event-data() -> ()  [unwired: 1 in, 6 out]
        n532 = Unbundle By Name(w1113) -> ("Label"=w1112:string)
        "Label" <- w1112
        n533 = case shown="\"Cuadriceps\"" w1112 {
          tunnel: [w1116 w1131 w1144 w1154 w1167 w1180 w1193 w1206 w1219 w1232 w1245 w1258] -> w1114
          tunnel: w1113 -> [w1127 w1140 w1153 w1166 w1179 w1192 w1205 w1218 w1231 w1244 w1257 w1258]
          tunnel: w1111 -> [w1118 w1130 w1143 w1155 w1169 w1182 w1194 w1208 w1221 w1234 w1247 _]
          tunnel: w1110 -> [w1117 w1129 w1142 w1156 w1168 w1181 w1195 w1207 w1220 w1233 w1246 _]
          frame "Cuadriceps" {
            n534 = Unbundle By Name(w1127) -> ("Cuadriceps"=w1119:i32)
            n535 = Greater Or Equal To 0?(x=w1119) -> (x >= 0?=w1124:bool)
            n536 = Less Or Equal?(x=w1119, y=100) -> (x <= y?=w1122:bool)
            n537 = Add(x=w1119, y=5) -> (x+y=w1126:i32)
            n538 = And(x=w1124, y=w1122) -> (x .and. y?=w1123:bool)
            n539 = Select(t=w1126, s=w1123, f=w1119) -> (s? t:f=w1120:i32)
            n540 = Bundle By Name(cluster=w1127, "Cuadriceps"=w1120, "Label"="Cuadriceps") -> (w1116:T1)
            n541 = Enqueue Element(queue=w1117, element=w1116, error in (no error)=w1118) -> ()  [unwired: 1 in, 3 out]
          }
          frame "Isquiotibiales" {
            n542 = Unbundle By Name(w1140) -> ("Isquiotibiales"=w1132:i32)
            n543 = Greater Or Equal To 0?(x=w1132) -> (x >= 0?=w1137:bool)
            n544 = Less Or Equal?(x=w1132, y=100) -> (x <= y?=w1135:bool)
            n545 = Add(x=w1132, y=5) -> (x+y=w1139:i32)
            n546 = And(x=w1137, y=w1135) -> (x .and. y?=w1136:bool)
            n547 = Select(t=w1139, s=w1136, f=w1132) -> (s? t:f=w1133:i32)
            n548 = Bundle By Name(cluster=w1140, "Isquiotibiales"=w1133, "Label"="Isquiotibiales") -> (w1131:T1)
            n549 = Enqueue Element(queue=w1129, element=w1131, error in (no error)=w1130) -> ()  [unwired: 1 in, 3 out]
          }
          frame "Gluteos" {
            n550 = Unbundle By Name(w1153) -> ("Gluteos"=w1145:i32)
            n551 = Greater Or Equal To 0?(x=w1145) -> (x >= 0?=w1150:bool)
            n552 = Less Or Equal?(x=w1145, y=100) -> (x <= y?=w1148:bool)
            n553 = Add(x=w1145, y=5) -> (x+y=w1152:i32)
            n554 = And(x=w1150, y=w1148) -> (x .and. y?=w1149:bool)
            n555 = Select(t=w1152, s=w1149, f=w1145) -> (s? t:f=w1146:i32)
            n556 = Bundle By Name(cluster=w1153, "Gluteos"=w1146, "Label"="Gluteos") -> (w1144:T1)
            n557 = Enqueue Element(queue=w1142, element=w1144, error in (no error)=w1143) -> ()  [unwired: 1 in, 3 out]
          }
          frame "Abdomen" {
            n558 = Unbundle By Name(w1166) -> ("Abdomen"=w1158:i32)
            n559 = Greater Or Equal To 0?(x=w1158) -> (x >= 0?=w1163:bool)
            n560 = Less Or Equal?(x=w1158, y=100) -> (x <= y?=w1161:bool)
            n561 = Add(x=w1158, y=5) -> (x+y=w1165:i32)
            n562 = And(x=w1163, y=w1161) -> (x .and. y?=w1162:bool)
            n563 = Select(t=w1165, s=w1162, f=w1158) -> (s? t:f=w1159:i32)
            n564 = Bundle By Name(cluster=w1166, "Abdomen"=w1159, "Label"="Abdomen") -> (w1154:T1)
            n565 = Enqueue Element(queue=w1156, element=w1154, error in (no error)=w1155) -> ()  [unwired: 1 in, 3 out]
          }
          frame "Lumbares" {
            n566 = Unbundle By Name(w1179) -> ("Lumbares"=w1171:i32)
            n567 = Greater Or Equal To 0?(x=w1171) -> (x >= 0?=w1176:bool)
            n568 = Less Or Equal?(x=w1171, y=100) -> (x <= y?=w1174:bool)
            n569 = Add(x=w1171, y=5) -> (x+y=w1178:i32)
            n570 = And(x=w1176, y=w1174) -> (x .and. y?=w1175:bool)
            n571 = Select(t=w1178, s=w1175, f=w1171) -> (s? t:f=w1172:i32)
            n572 = Bundle By Name(cluster=w1179, "Lumbares"=w1172, "Label"="Lumbares") -> (w1167:T1)
            n573 = Enqueue Element(queue=w1168, element=w1167, error in (no error)=w1169) -> ()  [unwired: 1 in, 3 out]
          }
          frame "Dorsales" {
            n574 = Unbundle By Name(w1192) -> ("Dorsales"=w1184:i32)
            n575 = Greater Or Equal To 0?(x=w1184) -> (x >= 0?=w1189:bool)
            n576 = Less Or Equal?(x=w1184, y=100) -> (x <= y?=w1187:bool)
            n577 = Add(x=w1184, y=5) -> (x+y=w1191:i32)
            n578 = And(x=w1189, y=w1187) -> (x .and. y?=w1188:bool)
            n579 = Select(t=w1191, s=w1188, f=w1184) -> (s? t:f=w1185:i32)
            n580 = Bundle By Name(cluster=w1192, "Dorsales"=w1185, "Label"="Dorsales") -> (w1180:T1)
            n581 = Enqueue Element(queue=w1181, element=w1180, error in (no error)=w1182) -> ()  [unwired: 1 in, 3 out]
          }
          frame "Trapecio" {
            n582 = Unbundle By Name(w1205) -> ("Trapecio"=w1197:i32)
            n583 = Greater Or Equal To 0?(x=w1197) -> (x >= 0?=w1202:bool)
            n584 = Less Or Equal?(x=w1197, y=100) -> (x <= y?=w1200:bool)
            n585 = Add(x=w1197, y=5) -> (x+y=w1204:i32)
            n586 = And(x=w1202, y=w1200) -> (x .and. y?=w1201:bool)
            n587 = Select(t=w1204, s=w1201, f=w1197) -> (s? t:f=w1198:i32)
            n588 = Bundle By Name(cluster=w1205, "Trapecio"=w1198, "Label"="Trapecio") -> (w1193:T1)
            n589 = Enqueue Element(queue=w1195, element=w1193, error in (no error)=w1194) -> ()  [unwired: 1 in, 3 out]
          }
          frame "Pectorales" {
            n590 = Unbundle By Name(w1218) -> ("Pectorales"=w1210:i32)
            n591 = Greater Or Equal To 0?(x=w1210) -> (x >= 0?=w1215:bool)
            n592 = Less Or Equal?(x=w1210, y=100) -> (x <= y?=w1213:bool)
            n593 = Add(x=w1210, y=5) -> (x+y=w1217:i32)
            n594 = And(x=w1215, y=w1213) -> (x .and. y?=w1214:bool)
            n595 = Select(t=w1217, s=w1214, f=w1210) -> (s? t:f=w1211:i32)
            n596 = Bundle By Name(cluster=w1218, "Pectorales"=w1211, "Label"="Pectorales") -> (w1206:T1)
            n597 = Enqueue Element(queue=w1207, element=w1206, error in (no error)=w1208) -> ()  [unwired: 1 in, 3 out]
          }
          frame "Biceps" {
            n598 = Unbundle By Name(w1231) -> ("Biceps"=w1223:i32)
            n599 = Greater Or Equal To 0?(x=w1223) -> (x >= 0?=w1228:bool)
            n600 = Less Or Equal?(x=w1223, y=100) -> (x <= y?=w1226:bool)
            n601 = Add(x=w1223, y=5) -> (x+y=w1230:i32)
            n602 = And(x=w1228, y=w1226) -> (x .and. y?=w1227:bool)
            n603 = Select(t=w1230, s=w1227, f=w1223) -> (s? t:f=w1224:i32)
            n604 = Bundle By Name(cluster=w1231, "Biceps"=w1224, "Label"="Biceps") -> (w1219:T1)
            n605 = Enqueue Element(queue=w1220, element=w1219, error in (no error)=w1221) -> ()  [unwired: 1 in, 3 out]
          }
          frame "Opcional" {
            n606 = Unbundle By Name(w1244) -> ("Opcional"=w1236:i32)
            n607 = Greater Or Equal To 0?(x=w1236) -> (x >= 0?=w1241:bool)
            n608 = Less Or Equal?(x=w1236, y=100) -> (x <= y?=w1239:bool)
            n609 = Add(x=w1236, y=5) -> (x+y=w1243:i32)
            n610 = And(x=w1241, y=w1239) -> (x .and. y?=w1240:bool)
            n611 = Select(t=w1243, s=w1240, f=w1236) -> (s? t:f=w1237:i32)
            n612 = Bundle By Name(cluster=w1244, "Opcional"=w1237, "Label"="Opcional") -> (w1232:T1)
            n613 = Enqueue Element(queue=w1233, element=w1232, error in (no error)=w1234) -> ()  [unwired: 1 in, 3 out]
          }
          frame "Master" {
            n614 = Unbundle By Name(w1257) -> ("Master"=w1249:i32)
            n615 = Greater Or Equal To 0?(x=w1249) -> (x >= 0?=w1254:bool)
            n616 = Less?(x=w1249, y=100) -> (x < y?=w1252:bool)
            n617 = Add(x=w1249, y=5) -> (x+y=w1256:i32)
            n618 = And(x=w1254, y=w1252) -> (x .and. y?=w1253:bool)
            n619 = Select(t=w1256, s=w1253, f=w1249) -> (s? t:f=w1250:i32)
            n620 = Bundle By Name(cluster=w1257, "Master"=w1250, "Label"="Master") -> (w1245:T1)
            n621 = Enqueue Element(queue=w1246, element=w1245, error in (no error)=w1247) -> ()  [unwired: 1 in, 3 out]
          }
          frame Default {
          }
        }
      }
      event "Remove Button": Value Change {
        n622 = event-data() -> ()  [unwired: 1 in, 6 out]
        n623 = Unbundle By Name(w1262) -> ("Label"=w1261:string)
        n624 = case shown="\"Cuadriceps\"" w1261 {
          tunnel: [w1264 w1275 w1284 w1294 w1304 w1314 w1325 w1334 w1344 w1354 w1364 w1374] -> w1263
          tunnel: w1262 -> [w1273 w1283 w1293 w1303 w1313 w1323 w1333 w1343 w1353 w1363 w1373 w1374]
          tunnel: w1260 -> [w1265 w1276 w1285 w1295 w1306 w1315 w1327 w1335 w1346 w1356 w1366 _]
          tunnel: w1259 -> [w1266 w1277 w1286 w1296 w1305 w1316 w1326 w1336 w1345 w1355 w1365 _]
          frame "Cuadriceps" {
            n625 = Unbundle By Name(w1273) -> ("Cuadriceps"=w1268:i32)
            n626 = Greater Than 0?(x=w1268) -> (x > 0?=w1270:bool)
            n627 = Subtract(x=w1268, y=5) -> (x-y=w1271:i32)
            n628 = Select(t=w1271, s=w1270, f=w1268) -> (s? t:f=w1269:i32)
            n629 = Bundle By Name(cluster=w1273, "Cuadriceps"=w1269, "Label"="Cuadriceps") -> (w1264:T1)
            n630 = Enqueue Element(queue=w1265, element=w1264, error in (no error)=w1266) -> ()  [unwired: 1 in, 3 out]
          }
          frame "Isquiotibiales" {
            n631 = Unbundle By Name(w1283) -> ("Isquiotibiales"=w1278:i32)
            n632 = Greater Than 0?(x=w1278) -> (x > 0?=w1280:bool)
            n633 = Subtract(x=w1278, y=5) -> (x-y=w1281:i32)
            n634 = Select(t=w1281, s=w1280, f=w1278) -> (s? t:f=w1279:i32)
            n635 = Bundle By Name(cluster=w1283, "Isquiotibiales"=w1279, "Label"="Isquiotibiales") -> (w1275:T1)
            n636 = Enqueue Element(queue=w1276, element=w1275, error in (no error)=w1277) -> ()  [unwired: 1 in, 3 out]
          }
          frame "Gluteos" {
            n637 = Unbundle By Name(w1293) -> ("Gluteos"=w1288:i32)
            n638 = Greater Than 0?(x=w1288) -> (x > 0?=w1290:bool)
            n639 = Subtract(x=w1288, y=5) -> (x-y=w1291:i32)
            n640 = Select(t=w1291, s=w1290, f=w1288) -> (s? t:f=w1289:i32)
            n641 = Bundle By Name(cluster=w1293, "Gluteos"=w1289, "Label"="Gluteos") -> (w1284:T1)
            n642 = Enqueue Element(queue=w1285, element=w1284, error in (no error)=w1286) -> ()  [unwired: 1 in, 3 out]
          }
          frame "Abdomen" {
            n643 = Unbundle By Name(w1303) -> ("Abdomen"=w1298:i32)
            n644 = Greater Than 0?(x=w1298) -> (x > 0?=w1300:bool)
            n645 = Subtract(x=w1298, y=5) -> (x-y=w1301:i32)
            n646 = Select(t=w1301, s=w1300, f=w1298) -> (s? t:f=w1299:i32)
            n647 = Bundle By Name(cluster=w1303, "Abdomen"=w1299, "Label"="Abdomen") -> (w1294:T1)
            n648 = Enqueue Element(queue=w1295, element=w1294, error in (no error)=w1296) -> ()  [unwired: 1 in, 3 out]
          }
          frame "Lumbares" {
            n649 = Unbundle By Name(w1313) -> ("Lumbares"=w1308:i32)
            n650 = Greater Than 0?(x=w1308) -> (x > 0?=w1310:bool)
            n651 = Subtract(x=w1308, y=5) -> (x-y=w1311:i32)
            n652 = Select(t=w1311, s=w1310, f=w1308) -> (s? t:f=w1309:i32)
            n653 = Bundle By Name(cluster=w1313, "Lumbares"=w1309, "Label"="Lumbares") -> (w1304:T1)
            n654 = Enqueue Element(queue=w1306, element=w1304, error in (no error)=w1305) -> ()  [unwired: 1 in, 3 out]
          }
          frame "Dorsales" {
            n655 = Unbundle By Name(w1323) -> ("Dorsales"=w1318:i32)
            n656 = Greater Than 0?(x=w1318) -> (x > 0?=w1320:bool)
            n657 = Subtract(x=w1318, y=5) -> (x-y=w1321:i32)
            n658 = Select(t=w1321, s=w1320, f=w1318) -> (s? t:f=w1319:i32)
            n659 = Bundle By Name(cluster=w1323, "Dorsales"=w1319, "Label"="Dorsales") -> (w1314:T1)
            n660 = Enqueue Element(queue=w1315, element=w1314, error in (no error)=w1316) -> ()  [unwired: 1 in, 3 out]
          }
          frame "Trapecio" {
            n661 = Unbundle By Name(w1333) -> ("Trapecio"=w1328:i32)
            n662 = Greater Than 0?(x=w1328) -> (x > 0?=w1330:bool)
            n663 = Subtract(x=w1328, y=5) -> (x-y=w1331:i32)
            n664 = Select(t=w1331, s=w1330, f=w1328) -> (s? t:f=w1329:i32)
            n665 = Bundle By Name(cluster=w1333, "Trapecio"=w1329, "Label"="Trapecio") -> (w1325:T1)
            n666 = Enqueue Element(queue=w1327, element=w1325, error in (no error)=w1326) -> ()  [unwired: 1 in, 3 out]
          }
          frame "Pectorales" {
            n667 = Unbundle By Name(w1343) -> ("Pectorales"=w1338:i32)
            n668 = Greater Than 0?(x=w1338) -> (x > 0?=w1340:bool)
            n669 = Subtract(x=w1338, y=5) -> (x-y=w1341:i32)
            n670 = Select(t=w1341, s=w1340, f=w1338) -> (s? t:f=w1339:i32)
            n671 = Bundle By Name(cluster=w1343, "Pectorales"=w1339, "Label"="Pectorales") -> (w1334:T1)
            n672 = Enqueue Element(queue=w1335, element=w1334, error in (no error)=w1336) -> ()  [unwired: 1 in, 3 out]
          }
          frame "Biceps" {
            n673 = Unbundle By Name(w1353) -> ("Biceps"=w1348:i32)
            n674 = Greater Than 0?(x=w1348) -> (x > 0?=w1350:bool)
            n675 = Subtract(x=w1348, y=5) -> (x-y=w1351:i32)
            n676 = Select(t=w1351, s=w1350, f=w1348) -> (s? t:f=w1349:i32)
            n677 = Bundle By Name(cluster=w1353, "Biceps"=w1349, "Label"="Biceps") -> (w1344:T1)
            n678 = Enqueue Element(queue=w1346, element=w1344, error in (no error)=w1345) -> ()  [unwired: 1 in, 3 out]
          }
          frame "Opcional" {
            n679 = Unbundle By Name(w1363) -> ("Opcional"=w1358:i32)
            n680 = Greater Than 0?(x=w1358) -> (x > 0?=w1360:bool)
            n681 = Subtract(x=w1358, y=5) -> (x-y=w1361:i32)
            n682 = Select(t=w1361, s=w1360, f=w1358) -> (s? t:f=w1359:i32)
            n683 = Bundle By Name(cluster=w1363, "Opcional"=w1359, "Label"="Opcional") -> (w1354:T1)
            n684 = Enqueue Element(queue=w1356, element=w1354, error in (no error)=w1355) -> ()  [unwired: 1 in, 3 out]
          }
          frame "Master" {
            n685 = Unbundle By Name(w1373) -> ("Master"=w1368:i32)
            n686 = Greater Than 0?(x=w1368) -> (x > 0?=w1370:bool)
            n687 = Subtract(x=w1368, y=5) -> (x-y=w1371:i32)
            n688 = Select(t=w1371, s=w1370, f=w1368) -> (s? t:f=w1369:i32)
            n689 = Bundle By Name(cluster=w1373, "Master"=w1369, "Label"="Master") -> (w1364:T1)
            n690 = Enqueue Element(queue=w1366, element=w1364, error in (no error)=w1365) -> ()  [unwired: 1 in, 3 out]
          }
          frame Default {
          }
        }
      }
      event "Slider": Value Change {
        n691 = event-data() -> ()  [unwired: 1 in, 6 out]
        n692 = Unbundle By Name(w1379) -> ("Label"=w1377:string)
        n693 = case shown="\"Cuadriceps\"" w1377 {
          tunnel: [w1381 w1387 w1393 w1399 w1405 w1411 w1417 w1423 w1429 w1435 w1441 w1447] -> w1380
          tunnel: w1379 -> [w1386 w1392 w1398 w1404 w1410 w1416 w1422 w1428 w1434 w1440 w1446 w1447]
          tunnel: "Slider" -> [w1385 w1391 w1397 w1403 w1409 w1415 w1421 w1427 w1433 w1439 w1445 _]
          tunnel: w1376 -> [w1382 w1389 w1395 w1401 w1406 w1413 w1419 w1425 w1431 w1437 w1443 _]
          tunnel: w1375 -> [w1383 w1388 w1394 w1400 w1407 w1412 w1418 w1424 w1430 w1436 w1442 _]
          frame "Cuadriceps" {
            n694 = Bundle By Name(cluster=w1386, "Cuadriceps"=w1385, "Label"="Cuadriceps") -> (w1381:T1)
            n695 = Enqueue Element(queue=w1383, element=w1381, error in (no error)=w1382) -> ()  [unwired: 1 in, 3 out]
          }
          frame "Isquiotibiales" {
            n696 = Bundle By Name(cluster=w1392, "Isquiotibiales"=w1391, "Label"="Isquiotibiales") -> (w1387:T1)
            n697 = Enqueue Element(queue=w1388, element=w1387, error in (no error)=w1389) -> ()  [unwired: 1 in, 3 out]
          }
          frame "Gluteos" {
            n698 = Bundle By Name(cluster=w1398, "Gluteos"=w1397, "Label"="Gluteos") -> (w1393:T1)
            n699 = Enqueue Element(queue=w1394, element=w1393, error in (no error)=w1395) -> ()  [unwired: 1 in, 3 out]
          }
          frame "Abdomen" {
            n700 = Bundle By Name(cluster=w1404, "Abdomen"=w1403, "Label"="Abdomen") -> (w1399:T1)
            n701 = Enqueue Element(queue=w1400, element=w1399, error in (no error)=w1401) -> ()  [unwired: 1 in, 3 out]
          }
          frame "Lumbares" {
            n702 = Bundle By Name(cluster=w1410, "Lumbares"=w1409, "Label"="Lumbares") -> (w1405:T1)
            n703 = Enqueue Element(queue=w1407, element=w1405, error in (no error)=w1406) -> ()  [unwired: 1 in, 3 out]
          }
          frame "Dorsales" {
            n704 = Bundle By Name(cluster=w1416, "Dorsales"=w1415, "Label"="Dorsales") -> (w1411:T1)
            n705 = Enqueue Element(queue=w1412, element=w1411, error in (no error)=w1413) -> ()  [unwired: 1 in, 3 out]
          }
          frame "Trapecio" {
            n706 = Bundle By Name(cluster=w1422, "Trapecio"=w1421, "Label"="Trapecio") -> (w1417:T1)
            n707 = Enqueue Element(queue=w1418, element=w1417, error in (no error)=w1419) -> ()  [unwired: 1 in, 3 out]
          }
          frame "Pectorales" {
            n708 = Bundle By Name(cluster=w1428, "Pectorales"=w1427, "Label"="Pectorales") -> (w1423:T1)
            n709 = Enqueue Element(queue=w1424, element=w1423, error in (no error)=w1425) -> ()  [unwired: 1 in, 3 out]
          }
          frame "Biceps" {
            n710 = Bundle By Name(cluster=w1434, "Biceps"=w1433, "Label"="Biceps") -> (w1429:T1)
            n711 = Enqueue Element(queue=w1430, element=w1429, error in (no error)=w1431) -> ()  [unwired: 1 in, 3 out]
          }
          frame "Opcional" {
            n712 = Bundle By Name(cluster=w1440, "Opcional"=w1439, "Label"="Opcional") -> (w1435:T1)
            n713 = Enqueue Element(queue=w1436, element=w1435, error in (no error)=w1437) -> ()  [unwired: 1 in, 3 out]
          }
          frame "Master" {
            n714 = Bundle By Name(cluster=w1446, "Master"=w1445, "Label"="Master") -> (w1441:T1)
            n715 = Enqueue Element(queue=w1442, element=w1441, error in (no error)=w1443) -> ()  [unwired: 1 in, 3 out]
          }
          frame Default {
          }
        }
      }
      event "Stop": Value Change {
        n716 = event-data() -> ()  [unwired: 1 in, 6 out]
      }
      event "Back": Value Change {
        n717 = event-data() -> ()  [unwired: 1 in, 6 out]
        n718 = Bundle By Name(cluster=w1452, "Label"="Back" ("Message")) -> (w1450:T1)
      }
      event "Master": Value Change {
        n719 = event-data() -> ()  [unwired: 1 in, 6 out]
        n720 = property on="Master" class="Bool (strict)"() -> ("Colors [4]"=w1456:cluster{u32, u32}[])  [unwired: 2 in, 2 out]
        n721 = Index Array(array=w1456) -> (element=w1459:cluster{u32, u32})  [unwired: 1 in]
        n722 = Bundle By Name(cluster=w1463, "Label"="Master" ("Message")) -> (w1461:T1)
        n723 = Unbundle(w1459) -> (w1458:u32, w1457:u32)
        n724 = case shown="True" "Master" {
          tunnel: [u32 16711680 ("Boolean Text.Text Colors:Text Color") u32 16448250 ("Boolean Text.Text Colors:Text Color")] -> w1460
          tunnel: w1458 -> [_ w1472]
          tunnel: w1457 -> [w1470 _]
          tunnel: w1456 -> [w1468 w1474]
          tunnel: [w1465 w1475] -> w1455
          frame False {
            n725 = Bundle("Boolean Text.Text Colors:Text Color"=u32 13816530, w1470) -> (w1467:T2)  [unwired: 1 in]
            n726 = Replace Array Subset(array=w1468, new element=w1467, index=0) -> (w1465:cluster{u32, u32}[])
          }
          frame True {
            n727 = Bundle(w1472, "Boolean Text.Text Colors:Text Color"=u32 16711680) -> (w1477:T3)  [unwired: 1 in]
            n728 = Replace Array Subset(array=w1474, new element=w1477, index=0) -> (w1475:cluster{u32, u32}[])
          }
        }
        n729 = property on="Master" class="Bool (strict)"("BoolText.TextColor"=w1460) -> ()  [unwired: 2 in, 2 out]
        n730 = property on="Master" class="Bool (strict)"("Colors [4]"=w1455) -> ()  [unwired: 2 in, 2 out]
        "Master" <- "Master"
      }
      event "Help": Value Change {
        n731 = event-data() -> ()  [unwired: 1 in, 6 out]
        n732 = call "Help.vi"() -> ()  [unwired: 11 in, 1 out]
      }
      event "Impulso": Value Change {
        n733 = event-data() -> ()  [unwired: 1 in, 6 out]
        n734 = call "Impulso.vi"() -> ("Parametros"=w1495:cluster{i32, i32, i32, i32, i32, dbl})  [unwired: 2 in]
        n735 = Unbundle(w1495) -> (w1488:i32, w1481:i32, w1485:dbl)  [unwired: 3 out]
        n736 = Bundle By Name(cluster=w1496, "Label"="Frecuencia" ("Message"), "Frecuencia"=w1488) -> (w1487:T1)
        n737 = Enqueue Element(queue=w1494, element=w1487, error in (no error)=w1493) -> (queue out=w1491:refnum<queue>, error out=w1492:errorcluster)  [unwired: 1 in, 1 out]
        n738 = Bundle By Name(cluster=w1487, "Label"="Ganancia", "Ganancia"=w1485) -> (w1484:T1)
        n739 = Enqueue Element(queue=w1491, element=w1484, error in (no error)=w1492) -> (queue out=w1489:refnum<queue>, error out=w1490:errorcluster)  [unwired: 1 in, 1 out]
        n740 = Bundle By Name(cluster=w1484, "Label"="Impulso", "Impulso"=w1481) -> (w1482:T1)
        n741 = Enqueue Element(queue=w1489, element=w1482, error in (no error)=w1490) -> ()  [unwired: 1 in, 3 out]
      }
      event "Reset": Value Change {
        n742 = event-data() -> ()  [unwired: 1 in, 6 out]
        n743 = Bundle By Name(cluster=w1548, "Label"="Cuadriceps" ("Message"), "Cuadriceps"=0) -> (w1541:T1)
        n744 = Enqueue Element(queue=w1547, element=w1541, error in (no error)=w1546) -> (queue out=w1544:refnum<queue>, error out=w1545:errorcluster)  [unwired: 1 in, 1 out]
        n745 = Bundle By Name(cluster=w1541, "Label"="Isquiotibiales", "Isquiotibiales"=0) -> (w1539:T1)
        n746 = Enqueue Element(queue=w1544, element=w1539, error in (no error)=w1545) -> (queue out=w1542:refnum<queue>, error out=w1543:errorcluster)  [unwired: 1 in, 1 out]
        n747 = Bundle By Name(cluster=w1539, "Label"="Gluteos", "Gluteos"=0) -> (w1530:T1)
        n748 = Enqueue Element(queue=w1542, element=w1530, error in (no error)=w1543) -> (queue out=w1533:refnum<queue>, error out=w1534:errorcluster)  [unwired: 1 in, 1 out]
        n749 = Bundle By Name(cluster=w1530, "Label"="Abdomen", "Abdomen"=0) -> (w1527:T1)
        n750 = Enqueue Element(queue=w1533, element=w1527, error in (no error)=w1534) -> (queue out=w1531:refnum<queue>, error out=w1532:errorcluster)  [unwired: 1 in, 1 out]
        n751 = Bundle By Name(cluster=w1527, "Label"="Lumbares", "Lumbares"=0) -> (w1524:T1)
        n752 = Enqueue Element(queue=w1531, element=w1524, error in (no error)=w1532) -> (queue out=w1520:refnum<queue>, error out=w1521:errorcluster)  [unwired: 1 in, 1 out]
        n753 = Bundle By Name(cluster=w1524, "Label"="Dorsales", "Dorsales"=0) -> (w1517:T1)
        n754 = Bundle By Name(cluster=w1517, "Label"="Trapecio", "Trapecio"=0) -> (w1514:T1)
        n755 = Enqueue Element(queue=w1520, element=w1517, error in (no error)=w1521) -> (queue out=w1518:refnum<queue>, error out=w1519:errorcluster)  [unwired: 1 in, 1 out]
        n756 = Enqueue Element(queue=w1518, element=w1514, error in (no error)=w1519) -> (queue out=w1511:refnum<queue>, error out=w1510:errorcluster)  [unwired: 1 in, 1 out]
        n757 = Bundle By Name(cluster=w1514, "Label"="Pectorales", "Pectorales"=0) -> (w1509:T1)
        n758 = Bundle By Name(cluster=w1509, "Label"="Biceps", "Biceps"=0) -> (w1504:T1)
        n759 = Enqueue Element(queue=w1511, element=w1509, error in (no error)=w1510) -> (queue out=w1505:refnum<queue>, error out=w1506:errorcluster)  [unwired: 1 in, 1 out]
        n760 = Enqueue Element(queue=w1505, element=w1504, error in (no error)=w1506) -> (queue out=w1500:refnum<queue>, error out=w1501:errorcluster)  [unwired: 1 in, 1 out]
        n761 = Bundle By Name(cluster=w1504, "Label"="Opcional", "Opcional"=0) -> (w1499:T1)
        n762 = Enqueue Element(queue=w1500, element=w1499, error in (no error)=w1501) -> ()  [unwired: 1 in, 3 out]
      }
      event "Start": Value Change {
        n763 = event-data() -> ()  [unwired: 1 in, 6 out]
        n764 = Bundle By Name(cluster=w1553, "Label"="Start" ("Message")) -> (w1552:T1)
        "Boolean" <- "Start"
      }
    }
  }
  n765 = VISA Close(VISA resource name=w10, error in (no error)=w11) -> (error out=→"error out 2":errorcluster)
  n766 = Release Queue(queue=w4, error in (no error)=w1) -> ()  [unwired: 1 in, 3 out]
  "error out" <- "error in (no error)"
